vi "CRYSignal Generator.vi"(0 "Output Level(RMS)":dbl(knob)=10.0 caption="输出电平(RMS)" min=0.0 max=0.0 step=0.01 scale=0.0..1.0 scale format="%.1p", 1 "Manual":bool=TRUE, 2 "Output Device":u32, 5 "EQ":bool caption="均衡", 7 "Signal Path":i16(ring) caption="信号通道" items=["Left", "Right"], 9 "Execution control":T2={"interactive"=TRUE, "displayed"=TRUE, "in a seq"=FALSE}, 11 "Mute":bool=TRUE, 12 "Hardware in":string, 13 "Cancel":bool, 14 "Calibration in":string) -> (4 "Freq Out":dbl=1000.0 caption="Actual Freq" format="%.2f", 6 "Amp Out":dbl=0.01 caption="Actual level" format="%.2f", 8 "Sigal generator setup Out":string="%#_6p", 10 "Channel Out":u32, 15 "Canceled?":bool)   [LabVIEW 2013]
uses:
  Typedef Control/CRYWaveFile Information Typedef.ctl
  Typedef Control/CRYHardware Channel Info.ctl
  SubVI/CRYMisc vis settings global.vi
  Calibration/SubVI/CRYCal Global.vi
  CRYMainGlobal.vi
  Task Sequence/CRYProject Run Control Global.vi
  <vilib>/Analysis/NI_AALPro.lvlib
  CRYSound.dll
panel:
  in  "OK1":bool caption="ok"
  out "Play noise":sgl[](array[numeric]) caption="play noise"
  out "Out level":dbl
  in  "asio finished":bool
  out "wave data out":i32[](array[numeric])
  in  "Dur_asio":dbl=1.0 caption="檬" min=0.01 format="%.1f"
  in  "isMain":bool
  out "Gen_Index":i32
  in  "asio inited":bool
  in  "nTime_Count":u32 caption="%"
  in  "BuffAmount":u32
  out "Buffer Amount":i32
  in  "buf_index":u32 caption="%"
  in  "asio start":bool
  out "change flag":bool
  in  "Asio OCI":u32 caption="%"
  in  "ASIO AMP":dbl=0.1 caption="%" min=0.0 format="%.1f"
  in  "ASIO FS":dbl=0.1 caption="%" min=0.0 format="%.1f"
  in  "Device Name":string
  in  "Audio Driver":u16
  out "error out":errorcluster
  out "rms R":dbl
  out "rms L":dbl
  in  "Sel Channel":u16(ring) caption="Peak Unit" items=["Left", "Right"]
  out "Load Test":bool
  out "Configure Data":string
  out "Set Configure":bool
  out "lin2":bool
  out "lin1":bool
  out "log2":bool
  out "log1":bool
  out "Menu":bool=TRUE
  out "VI nID":i32
  out "Title nID":i32
  out "StateOut":bool=TRUE
  out "Error Output":errorcluster
  out "Wave L":dbl caption="Wave RMS" format="%0.2f"
  in  "ReMake Flg":bool
  in  "Play Sine Wave:":i32(slide) caption="播放正弦信号"
  out "noise":sgl[](array[numeric])
  out "Byte num":u32
  out "wave info":T1={"total number of samples/ch"=16, "total byte number"=2, "Time DBL"=0.0, "format str"="", "Time Str"="", "peak FSD"=0.0, "rms FSD"=0.0, "peak %FSD"=0.0, "rms %FSD"=0.0, "rms"=0.0, "Channel Number"=0, "rms L"=0.0, "rms R"=0.0}
  in  "Fs":u32=44100 caption="Sampling Frequency"
  in  "BitDepth":u32=16
  in  "ntaskID":u32
  in  "Max(Hz)":dbl=1.0 caption="最大(Hz)" min=1.0 step=1.0 format="%#.4p"
  in  "Min (Hz)":dbl=20.0 caption="最小(Hz)" min=1.0 max=20948.0 format="%#.4p"
  in  "Duration(s)":dbl=1.0 caption="时间(秒)" min=0.0 max=1000.0 step=1.0 format="%#.3p"
  out "Time":string
  out "stereo":string
  out "RMS":dbl format="%.4g"
  out "Peak":dbl caption="最大值" format="%_6f"
  in  "RMS Unit":u16(ring) items=["dB FSD", "%FSD"]
  in  "Peak Unit":u16(ring) items=["dB FSD", "%FSD"]
  in  "mute flash":bool
  in  "sine ol min":dbl=0.1 caption="V" min=0.0 format="%.3f"
  in  "sine ol max":dbl=0.1 caption="V" min=0.0 format="%.3f"
  in  "sine ol log":bool
  in  "wav ol log":bool
  in  "wav ol max":dbl=0.1 caption="V" min=0.0 format="%.3f"
  in  "wav ol min":dbl=0.1 caption="V" min=0.0 format="%.3f"
  in  "Duration":dbl=1.0 caption="秒" min=0.01 format="%.1f"
  in  "Signal Type":i32(ring) caption="信号类型" items=["正弦波", "wav", "粉红噪声", "白噪声"]
  in  "Wave path":string caption="波文件路径"
  in  "Wave play mode":i32(slide) caption="播放波文件"
  in  "n times":i32=1 caption="N次" min=1
  in  "wav level":dbl=0.1 caption="%" min=0.0 format="%.1f"
  in  "sine level":dbl=0.1 caption="V" min=0.0 format="%.3p"
  in  "freq lin/log":bool
  in  "level lin/log":bool
  in  "close at end":bool
  in  "dB":dbl=-40.0 min=-1000.0 max=1000.0 step=0.1 format="%.1f"
  out "unit2":string="V"
  out "Error":u32
  in  "Sweep Rate":dbl=1.0 caption="Octave/s" min=0.1 step=0.01 format="%.2f"
  in  "Quadrature":bool
  in  "Sensitivity":dbl=1.0 min=0.1 step=0.01 format="%.6f"
  in  "Frequency":dbl(knob)=1000.0 caption="频率" min=10.0 max=20948.0 step=1.0 scale=20.0..20000.0
  out "mute border":bool
  in  "cont":bool=TRUE
  in  "Vp Out":dbl=2.6 min=0.1 step=0.01 format="%.2f"
  out "unit1":string="Hz"
  in  "Browse":bool
  in  "start":bool
  in  "stop":bool
  in  "OK":bool caption="ok"
  in  "cancel2":bool
  in  "1 kHz":bool
  in  "Equalization Out":cluster{"Hz":dbl, dbl, "Deg":dbl}[](array[cluster])=[{"Hz"=1.0, 1.0, "Deg"=0.0}, {"Hz"=20000.0, 1.0, "Deg"=0.0}] {"Deg" format="%.2f"; "?" format="%.2f"; "Hz" format="%.2f"}
  in  "dB ref.":dbl=1.0 min=0.01 step=0.01 format="%.6f"
  in  "prefix Out":string
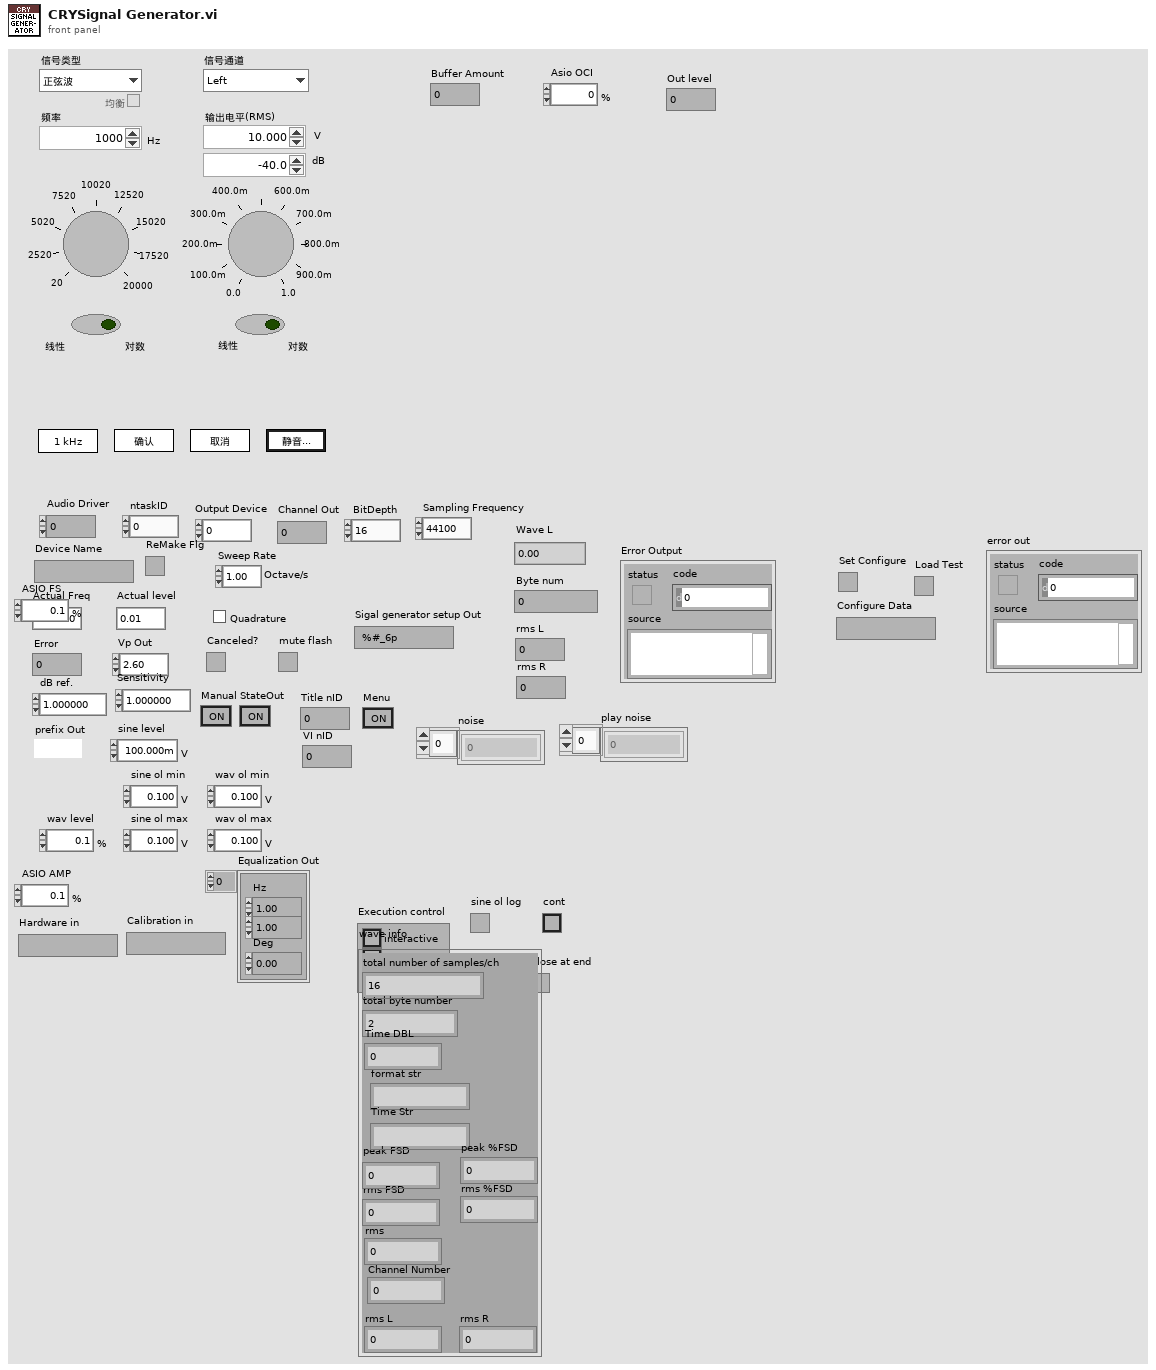
[diagram p1: front panel]
types:
  T1 = typedef "CRYWaveFile Information Typedef.ctl" = cluster{"total number of samples/ch":u32, "total byte number":u32, "Time DBL":dbl, "format str":string, "Time Str":string, "peak FSD":dbl, "rms FSD":dbl, "peak %FSD":dbl, "rms %FSD":dbl, "rms":dbl, "Channel Number":u16, "rms L":dbl, "rms R":dbl}
  T2 = cluster{"interactive":bool, "displayed":bool, "in a seq":bool}
  T3 = enum32{"Invalid", "Default", "Floating", "Floating/Auto-Hide", "Modal"}
  T4 = cluster{"wav play mode":i32, "start":bool, "Output Level(RMS)":dbl, "Output Level(dB)":dbl, "level lin/log":bool}
  T5 = cluster{"wav init":bool, "halt now":bool, "exit":bool, "dll done":bool, "called":bool, "changed":bool, "Hardware":i32}
  T6 = typedef "CRYCalibration All Cluster.ctl" = cluster{"Calibration 2D":T7[], "Help":string, "Tab Value":i32, "Input Signal Type":string, "Output Signal Type":string}
  T7 = typedef "CRYCalibration 2DCluster.ctl" = cluster{"Calibration":T8, "Corr Curve":T9, "EQ Curve":T9, "Sens Curve":T9}
  T8 = typedef "CRYCalibration Cluster.ctl" = cluster{"Calibration Step Name":string, "Device":string, "Correction Curve Name":string, "Equalization Curve Name":string, "Sensitivity Curve Name":string, "Corr Folder and File":string, "EQ Folder and File":string, "Sens Folder and File":string, "Corr Step size":u16, "EQ Step size":u16, "Input":bool, "Last Cal Date (sec)":timestamp, "Cha Name":string, "Corr Curve Found":bool, "EQ Curve Found":bool, "Sens Curve Found":bool, "Signal Type":string, "Calibrated Device":string, "Hz":u32}
  T9 = typedef "CRYData Cluster.ctl" = cluster{"Name":string, "Curve":cluster{"x":dbl, "y":dbl, "z":dbl}[], "X data":u16, "Y data":u16, "Z data":u16, "X axis":u16, "Y axis":u16, "Z axis":u16, "X unit":string, "Y unit":string, "Z unit":string, "X dB ref":dbl, "Y dB ref":dbl, "Z dB ref":dbl, "single val":bool, "protected":bool, "display X":bool, "display Y":bool, "display Z":bool, "Test Info":string, "Step No.":i32, "Plot Settings":cluster{"Color":u32, "Interpolation":u8, "Point Style":u8, "Line Style":u8, "Point Color":u32, "Line Width":u8, "Bar Plot Style":u8, "Fill To":i16}, "AutoProtect":bool}
  T10 = enum8{"Enabled", "Disabled", "Disabled and Grayed Out"}
  T11 = cluster{"gen'r mode":i32, "frequency":u32, "output level":dbl, "wave path":string, "wav play mode":i32, "duration":dbl, "n times":i32, "channel":i32, "wav level":dbl, "EQ":bool, "f knob log":bool, "f knob low":dbl, "f knob high":dbl, "ol knob log":bool, "ol knob low":dbl, "ol knob high":dbl, "Lin Display Prefs":string, "dB Display Prefs":string, "Duration noise":dbl, "Min freq noise":dbl, "Max freq noise":dbl, "Signal Type":string, "Play Sine Wave":i32}
  T12 = typedef "CRYHardware Channel Info.ctl" = cluster{"ID":i32, "Name":string, "Digital":bool, "Input":bool, "Device Name":string, "Hardware Ch ID":u8, "Vmax (V)":dbl, "Latency (samples)":dbl, "Sampling Rate (Hz)":u32, "Bit Depth":u32, "Anti-aliasing Factor (%fs)":sgl, "DAQmx Channel":tag, "term config":i32, "Coupling":i32, "IEPE en":bool, "ASIOChannel Name":string, "Audio Driver":u16, "ASIOChannel Index":u8}
  T13 = enum16{"sine", "cosine", "triangle", "square", "sawtooth", "increasing ramp", "decreasing ramp"}
  T14 = cluster{"Wave play mode":i32, "start":bool, "Output Level(RMS)":dbl, "dB":dbl, "level lin/log":bool}
  T15 = cluster{"Level Type":u16, "Vp Out":dbl, "Output Level(RMS)":dbl}
  T16 = cluster{"Gen Idx":i32, "Chn Idx":i32, "Data":sgl[]}[]
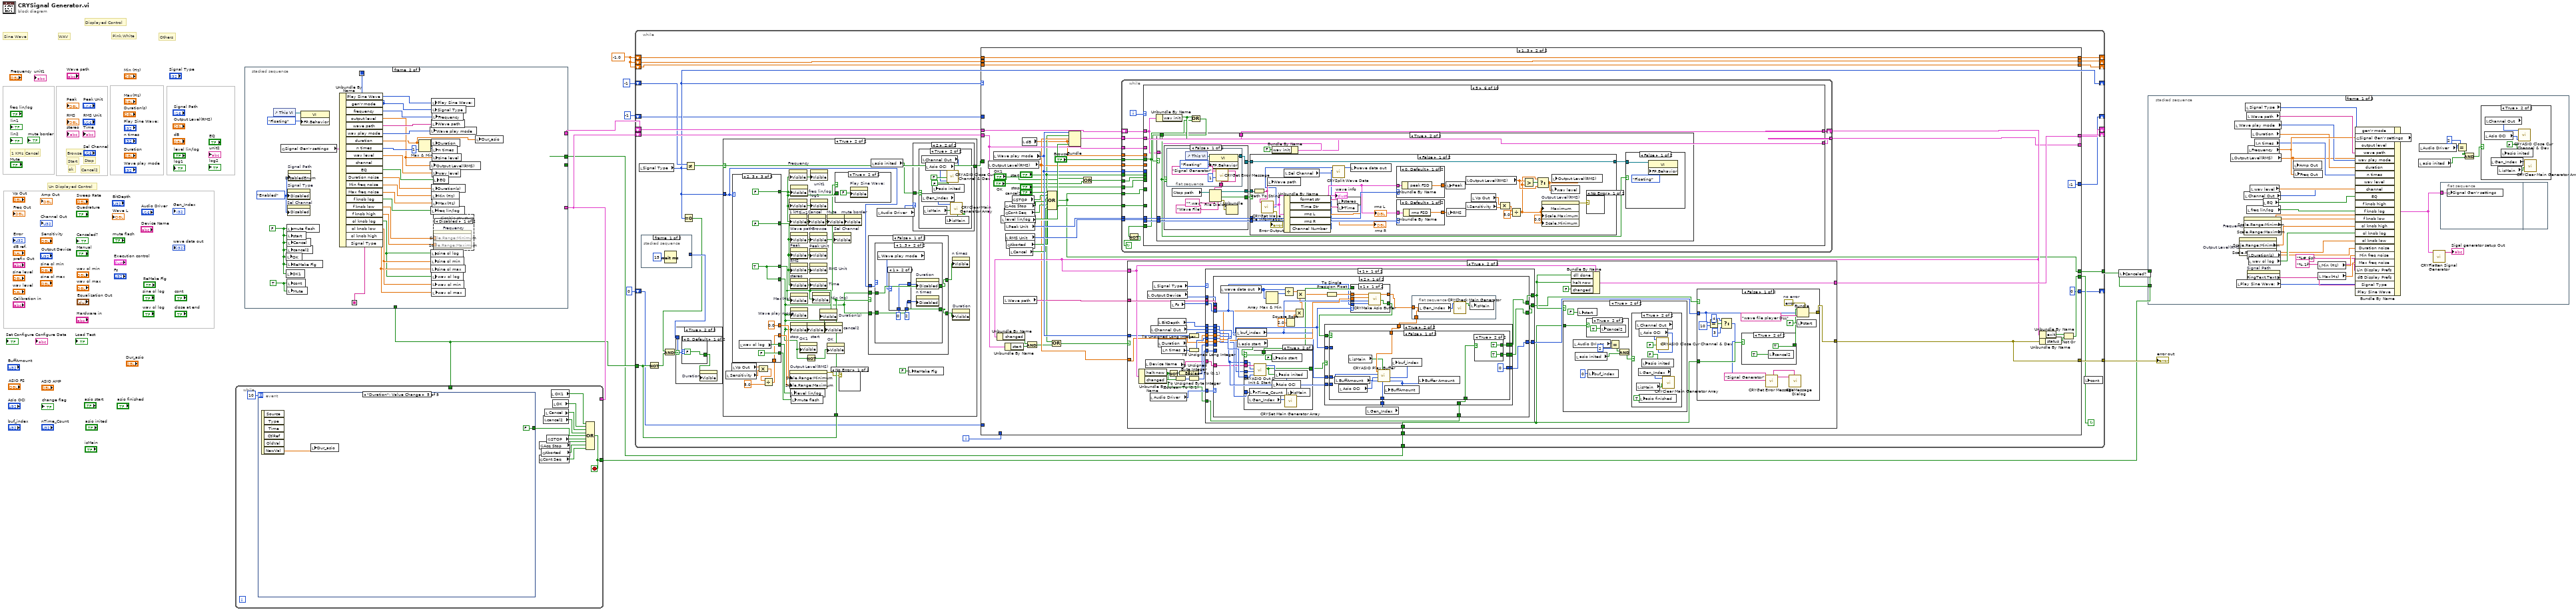
[diagram p0: block diagram]
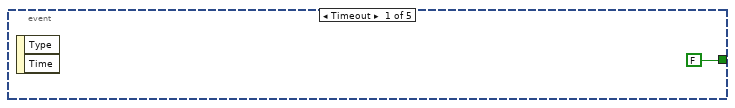
[diagram p2: hidden frame]
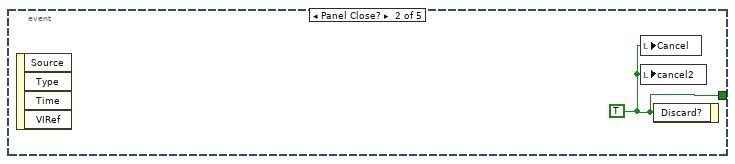
[diagram p3: hidden frame]
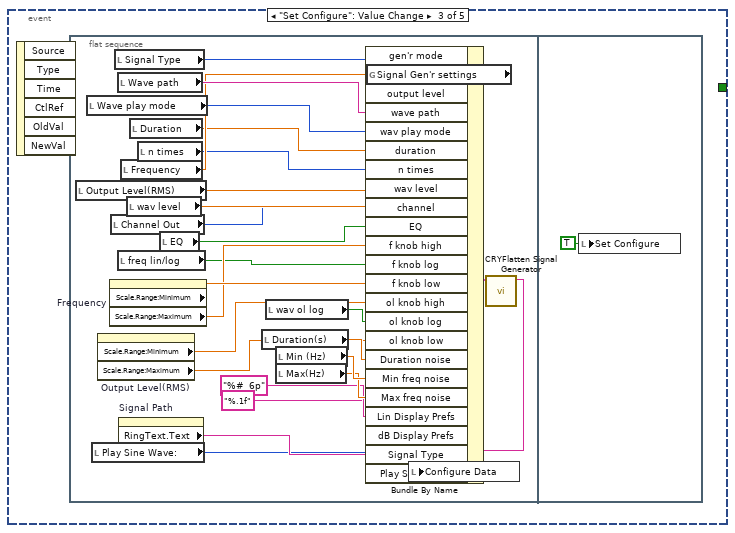
[diagram p4: hidden frame]
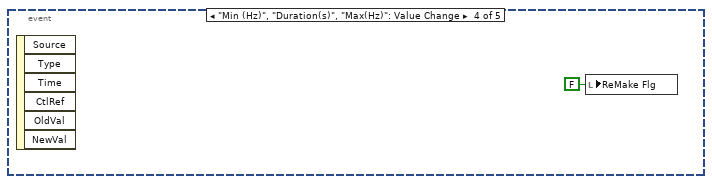
[diagram p5: hidden frame]
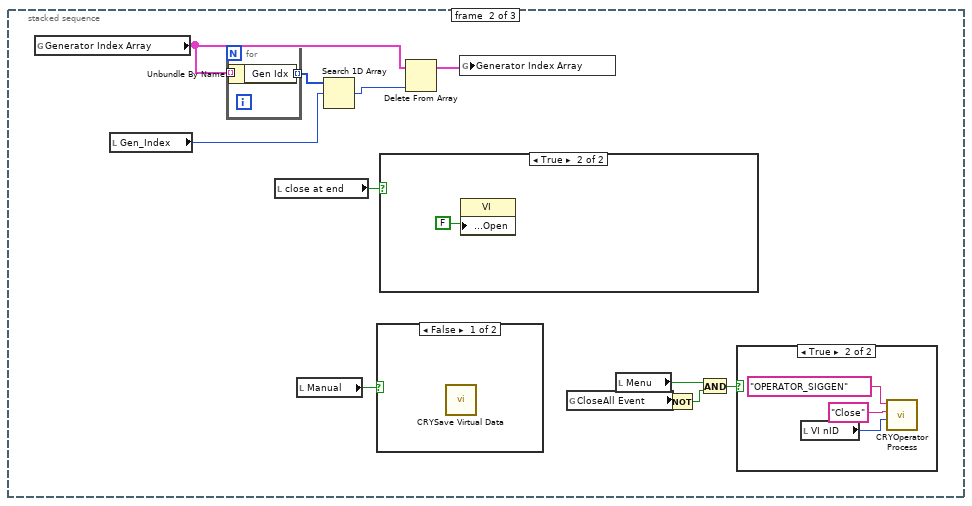
[diagram p7: hidden frame]
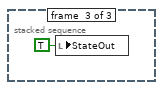
[diagram p11: hidden frame]
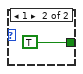
[diagram p13: hidden frame]
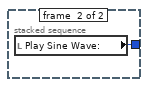
[diagram p14: hidden frame]
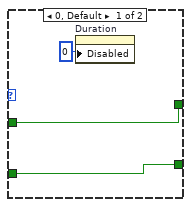
[diagram p19: hidden frame]
diagram:
  w1 = -1.0 ("Frequency")
  # "Others"
  # "WAV"
  # "Pink,White"
  # "Sine Wave"
  # "Un Displayed Control"
  # "Displayed Control"
  # "ok"
  # "Cancel2"
  # "Stop"
  # "Start"
  # "Browse"
  # "Cancel"
  # "1 KHz"
  n1 = stacked-sequence {
    seq-local: [_ w45 _ _ _ _ _] -> [_ _ _ w124 _ _ _]
    seq-local: [_ w41 _ _ _ _ _] -> [_ _ w66 _ _ _ _]
    tunnel: [_ _ _ w129 _ _ _] -> _
    tunnel: [_ _ _ w121 _ _ _] -> w4
    tunnel: [_ _ _ _ _ w170 _] -> w9
    tunnel: [_ _ _ _ _ T4 {"wav play mode"=-1, "start"=FALSE, "Output Level(RMS)"=0.0, "Output Level(dB)"=0.0, "level lin/log"=FALSE} _] -> w8
    tunnel: [_ _ _ w125 _ _ _] -> w7
    frame #0 {
      w16 = FALSE ("StateOut")
      n2 = call "CRYMake Generator Index.vi"() -> ("Gen_Index"=w12:i32)  [unwired: 11 in]
      n3 = local write "Set Configure"(w16) -> ()
      n4 = global read "CRYMisc vis settings global.vi" "Menu?"() -> (w21:bool)
      "Menu" <- w21
      n5 = local write "Gen_Index"(w12) -> ()
      n6 = call "CRYGet Window Title Message.vi"("No"=0 ("Error No"), "Kind"="Signal Generator") -> ("Multibyte String"=w19:string)  [unwired: 4 in, 5 out]
      n7 = case shown="True" w21 {
        tunnel: w19 -> [w24 w31]
        tunnel: [w24 w30] -> w18
        tunnel: [w23 w25] -> w13
        frame False {
          n8 = control-ref of="This VI"() -> (w22:refnum<vi>)
          n9 = call "CRYSet Signal Generator Front Panel.vi"("Vi Ref in"=w22) -> ()  [unwired: 10 in, 1 out]
          n10 = local read "Calibration in"() -> (w23:string)
        }
        frame True {
          n11 = global read "CRYMisc vis settings global.vi" "Execution control"() -> (w27:T2)
          n12 = global read "CRYMisc vis settings global.vi" "Temp Title nID"() -> (w32:i32)
          "Title nID" <- w32
          n13 = global read "CRYMisc vis settings global.vi" "Temp VI nID"() -> (→"VI nID":i32)
          n14 = global read "CRYMisc vis settings global.vi" "Manual"() -> (w34:bool)
          n15 = global read "CRYMisc vis settings global.vi" "Mute"() -> (w35:bool)
          n16 = call "CRYGet Current HC Steps.vi"() -> ("Calibration setup flattened Out"=w25:string, "Hardware setup flattened Out"=w26:string)  [unwired: 10 out]
          n17 = local write "Calibration in"(w25) -> ()
          n18 = local write "Hardware in"(w26) -> ()
          n19 = Number To Decimal String(number=w32) -> (decimal integer string=w29:string)  [unwired: 1 in]
          n20 = local write "Execution control"(w27) -> ()
          n21 = local write "Manual"(w34) -> ()
          n22 = local write "Mute"(w35) -> ()
          n23 = Concatenate Strings(w31, "-" ("string"), w29) -> (w30:string)
        }
      }
      n24 = property class="VI"("Front Panel.Title"=w18) -> ()  [unwired: 2 in, 2 out]
      n25 = call "CRYUnflatten Calibration 2D.vi"("Flattened Calibration"=w13) -> ("Calibration Step Out"=w14:T6)  [unwired: 8 in, 2 out]
      n26 = call "CRYGet Calibrated Device Name.vi"("Calibration"=w14) -> ("O_Signal Type Out"=w15:string[])  [unwired: 7 in, 7 out]
      n27 = property on="Signal Path" class="Ring (strict)"("Strings []"=w15) -> ()  [unwired: 2 in, 2 out]
      "StateOut" <- w16
    }
    frame #1 {
      w37 = T10."Enabled" ("Disabled")
      w44 = TRUE ("cont")
      w36 = FALSE ("Mute")
      n28 = control-ref of="This VI"() -> (w43:refnum<vi>)
      n29 = global read "CRYMisc vis settings global.vi" "Signal Gen'r settings"() -> (w53:T11)
      n30 = local write "OK"(w36) -> ()
      n31 = local write "OK1"(w36) -> ()
      n32 = local write "mute flash"(w36) -> ()
      n33 = local write "start"(w36) -> ()
      n34 = local write "Cancel"(w36) -> ()
      n35 = local write "cancel2"(w36) -> ()
      n36 = local write "ReMake Flg"(w36) -> ()
      n37 = local write "cont"(w44) -> ()
      n38 = local write "Mute"(w44) -> ()
      n39 = property on="Signal Type" class="Ring (strict)"("Disabled"=w37) -> ()  [unwired: 2 in, 2 out]
      n40 = property on="Sel Channel" class="Ring (strict)"("Disabled"=w37) -> ()  [unwired: 2 in, 2 out]
      n41 = property on="Signal Path" class="Ring (strict)"("DisabledEnum"=w37) -> ()  [unwired: 2 in, 2 out]
      n42 = property class="VI"(reference=w43, "FP.Behavior"=T3."Floating" ("Front Panel Window:Behavior")) -> ()  [unwired: 1 in, 2 out]
      n43 = Unbundle By Name(w53) -> ("Play Sine Wave"=w40:i32, "gen'r mode"=w45:i32, "frequency"=w58:u32, "output level"=w46:dbl, "wave path"=w60:string, "wav play mode"=w59:i32, "duration"=w38:dbl, "n times"=w61:i32, "wav level"=w57:dbl, "EQ"=w56:bool, "Duration noise"=w39:dbl, "Min freq noise"=w55:dbl, "Max freq noise"=w54:dbl, "f knob log"=w47:bool, "f knob low"=w48:dbl, "f knob high"=w49:dbl, "ol knob log"=w50:bool, "ol knob low"=w52:dbl, "ol knob high"=w51:dbl, "Signal Type"=w41:string)  [unwired: 1 out]
      n44 = Max & Min(x=1, y=w61) -> (max(x,y)=w62:i32)  [unwired: 1 out]
      n45 = local write "Wave play mode"(w59) -> ()
      n46 = local write "Output Level(RMS)"(w46) -> ()
      n47 = local write "freq lin/log"(w47) -> ()
      n48 = local write "sine ol log"(w50) -> ()
      n49 = local write "sine ol min"(w52) -> ()
      n50 = local write "sine ol max"(w51) -> ()
      n51 = local write "Play Sine Wave:"(w40) -> ()
      n52 = local write "Signal Type"(w45) -> ()
      n53 = local write "wav ol log"(w50) -> ()
      n54 = local write "wav ol min"(w52) -> ()
      n55 = local write "Wave path"(w60) -> ()
      n56 = local write "Duration"(w38) -> ()
      n57 = local write "Duration(s)"(w39) -> ()
      n58 = local write "Min (Hz)"(w55) -> ()
      n59 = local write "wav ol max"(w51) -> ()
      n60 = local write "Frequency"(w58) -> ()
      n61 = local write "n times"(w62) -> ()
      n62 = local write "sine level"(w46) -> ()
      n63 = local write "wav level"(w57) -> ()
      n64 = local write "Max(Hz)"(w54) -> ()
      n65 = local write "EQ"(w56) -> ()
      n66 = disable-structure shown="Disabled" {
        disable-tunnel: w49 -> [w65 _]
        disable-tunnel: w48 -> [w64 _]
        frame Disabled {
          n67 = property on="Frequency" class="Knob (strict)"("Scale.Range:Minimum"=w64, "Scale.Range:Maximum"=w65) -> ()  [unwired: 2 in, 2 out]
        }
        frame Enabled {
        }
      }
      n68 = local write "Dur_asio"(w38) -> ()
    }
    frame #2 {
      # "Initialize"
      n69 = local read "Manual"() -> (w67:bool)
      n70 = case shown="False" w67 {
        tunnel: w66 -> [w78 _]
        frame False {
          n71 = global read "CRYCal Global.vi" "Calibrate"() -> (w73:bool)
          n72 = local read "Calibration in"() -> (w74:string)
          n73 = local read "Hardware in"() -> (w75:string)
          n74 = case shown="False" w73 {
            tunnel: w78 -> [w89 _]
            tunnel: [w92 w107] -> w77
            tunnel: w75 -> [w91 w109]
            tunnel: w74 -> [w90 w108]
            tunnel: [w86 w106] -> w76
            frame False {
              n75 = call "CRYGet Hardware Info From Signal Type.vi"("Calibration In"=w90, "Hardware In"=w91, "Signal Type"=w89, "In/Out?"=FALSE) -> ("Exist?"=w94:bool, "Channel Info Out"=w93:T12)  [unwired: 5 in, 1 out]
              n76 = property on="Signal Path" class="Ring (strict)"() -> ("Strings []"=w88:string[])  [unwired: 2 in, 2 out]
              n77 = case shown="False" w94 {
                tunnel: w93 -> [_ w102]
                tunnel: [w97 w102] -> w92
                tunnel: w91 -> [w100 _]
                tunnel: w90 -> [w99 _]
                tunnel: w89 -> [_ w101]
                tunnel: [w96 w101] -> w87
                frame False {
                  w96 = "Direct Out 1" ("Signal Type")
                  n78 = call "CRYGet Hardware Info From Signal Type.vi"("Calibration In"=w99, "Hardware In"=w100, "Signal Type"=w96, "In/Out?"=FALSE) -> ("Channel Info Out"=w97:T12)  [unwired: 5 in, 2 out]
                }
                frame True {
                }
              }
              n79 = Search 1D Array(1D array=w88, element=w87) -> (index of element=w86:i32)  [unwired: 1 in]
            }
            frame True {
              n80 = global read "CRYCal Global.vi" "Signal Type Out"() -> (w106:u16)
              n81 = property on="Signal Path" class="Ring (strict)"() -> ("Strings []"=w105:string[])  [unwired: 2 in, 2 out]
              n82 = Index Array(array=w105, index=w106) -> (element=w103:string)
              n83 = call "CRYGet Hardware Info From Signal Type.vi"("Calibration In"=w108, "Hardware In"=w109, "Signal Type"=w103, "In/Out?"=FALSE) -> ("Channel Info Out"=w107:T12)  [unwired: 5 in, 2 out]
            }
          }
          n84 = local write "buf_index"(u32 0 ("buf_index")) -> ()
          n85 = Unbundle By Name(w77) -> ("ID"=w79:i32, "Hardware Ch ID"=w69:u8, "Vmax (V)"=w72:dbl, "Sampling Rate (Hz)"=w80:u32, "Bit Depth"=w81:u32, "Audio Driver"=w68:u16, "Device Name"=w71:string)
          n86 = local write "Signal Path"(w76) -> ()
          n87 = local write "Device Name"(w71) -> ()
          n88 = local write "Output Device"(w79) -> ()
          n89 = local write "Channel Out"(w69) -> ()
          n90 = local write "BitDepth"(w81) -> ()
          n91 = local write "Vp Out"(w72) -> ()
          n92 = local write "Fs"(w80) -> ()
          n93 = case shown="0, Default" w68 {
            tunnel: w69 -> [_ w85]
            frame 0, Default {
              n94 = local read "Gen_Index"() -> (w83:i32)
              n95 = call "CRYUpdate Generator Index.vi"("Chn Idx"=-1, "Gen_Index"=w83) -> ()  [unwired: 9 in]
            }
            frame 2 {
              n96 = local read "Gen_Index"() -> (w84:i32)
              n97 = call "CRYUpdate Generator Index.vi"("Chn Idx"=w85, "Gen_Index"=w84) -> ()  [unwired: 9 in]
            }
          }
          n98 = local write "Audio Driver"(w68) -> ()
        }
        frame True {
          w110 = T12[] [{"ID"=1, "Name"="Left", "Digital"=FALSE, "Input"=FALSE, "Device Name"="Card", "Hardware Ch ID"=0, "Vmax (V)"=2.6, "Latency (samples)"=67.0, "Sampling Rate (Hz)"=44100, "Bit Depth"=16, "Anti-aliasing Factor (%fs)"=44100.0, "DAQmx Channel"="", "term config"=0, "Coupling"=0, "IEPE en"=FALSE, "ASIOChannel Name"="", "Audio Driver"=0, "ASIOChannel Index"=0}, {"ID"=1, "Name"="Right", "Digital"=FALSE, "Input"=FALSE, "Device Name"="Card", "Hardware Ch ID"=1, "Vmax (V)"=2.6, "Latency (samples)"=67.0, "Sampling Rate (Hz)"=44100, "Bit Depth"=16, "Anti-aliasing Factor (%fs)"=44100.0, "DAQmx Channel"="", "term config"=0, "Coupling"=0, "IEPE en"=FALSE, "ASIOChannel Name"="", "Audio Driver"=0, "ASIOChannel Index"=0}] ("I_channel Info Out")
          n99 = call "CRYGet Channel Array.vi"("Channel Array"=w110) -> ("O_Channel Name Out"=w114:string[])  [unwired: 10 out]
          n100 = property on="Signal Path" class="Ring (strict)"("Strings []"=w114) -> ()  [unwired: 2 in, 2 out]
          n101 = Index Array(array=w110, index=1) -> (element=w120:T12)
          n102 = Unbundle By Name(w120) -> ("ID"=w118:i32, "Hardware Ch ID"=w119:u8)
          n103 = local write "Output Device"(w118) -> ()
          n104 = property on="Play Sine Wave:" class="Slide (strict)"("Visible"=FALSE) -> ()  [unwired: 2 in, 2 out]
          n105 = local write "Channel Out"(w119) -> ()
          n106 = local write "Vp Out"(2.6 ("Vmax (V)")) -> ()
          n107 = local write "BitDepth"(u32 16 ("BitDepth")) -> ()
          n108 = global write "CRYMainGlobal.vi" "STOP"(FALSE ("STOP")) -> ()
          n109 = local write "Fs"(u32 44100 ("Sampling Frequency")) -> ()
        }
      }
    }
    frame #3 {
      # "(formerly always displayed panel in continuous-play mode)"
      n110 = local read "Execution control"() -> (w127:T2)
      n111 = local read "Wave play mode"() -> (w126:i32)
      n112 = Unbundle By Name(w127) -> ("in a seq"=w121:bool, "interactive"=w125:bool, "displayed"=w132:bool)
      n113 = Equal To 0?(x=w126) -> (x = 0?=w128:bool)
      n114 = Greater Than 0?(x=w124) -> (x > 0?=w123:bool)
      n115 = case shown="False" w121 {
        frame False {
          w133 = 0 items=["Continuously", "for Duration"] ("Play Sine Wave:")
          n116 = local write "Play Sine Wave:"(w133) -> ()
        }
        frame True {
        }
      }
      n117 = property class="VI"() -> ("Front Panel Window:Open"=w122:bool)  [unwired: 2 in, 2 out]
      n118 = case shown="False" w123 {
        tunnel: w121 -> [w135 w136]
        frame False {
          n119 = Not(x=w135) -> (.not. x?=w134:bool)
          n120 = local write "Mute"(w134) -> ()
        }
        frame True {
          n121 = local write "start"(w136) -> ()
        }
      }
      n122 = Compound Arithmetic op=OR(invert w121, w128) -> (w129:bool)
      n123 = Or(x=w125, y=w132) -> (x .or. y?=w131:bool)
      n124 = Compound Arithmetic op=AND(w131, invert w122) -> (w130:bool)
      n125 = case shown="True" w131 {
        tunnel: w131 -> [_ w137]
        tunnel: w130 -> [_ _]
        frame False {
        }
        frame True {
          n126 = flat-sequence {
            tunnel: w137 -> [w138]
            frame #0 {
              n127 = property class="VI"("Front Panel Window:Open"=w138) -> ()  [unwired: 2 in, 2 out]
            }
            frame #1 {
              n128 = Wait (ms)(milliseconds to wait=u32 150) -> ()  [unwired: 1 out]
            }
          }
        }
      }
      n129 = local write "close at end"(w130) -> ()
    }
    frame #4 {
      n130 = local read "Manual"() -> (w140:bool)
      n131 = case shown="False" w140 {
        frame False {
          n132 = property on="Signal Path" class="Ring (strict)"() -> ("RingText.Text"=w147:string)  [unwired: 2 in, 2 out]
          n133 = call "CRYGet Current Calibration Info.vi"("Is Input?"=FALSE, "Signal Type Name"=w147) -> ("Calibration All Cluster"=w146:T7)  [unwired: 9 out]
          n134 = Unbundle By Name(w146) -> ("EQ Curve"=w154:T9, "Sens Curve"=w156:T9)
          n135 = Unbundle By Name(w156) -> ("Curve"=w158:cluster{"x":dbl, "y":dbl, "z":dbl}[], "Y unit"=w142:string, "Y dB ref"=w149:dbl)
          n136 = Unbundle By Name(w154) -> ("Curve"=w155:cluster{"x":dbl, "y":dbl, "z":dbl}[])  [unwired: 1 out]
          n137 = global read "CRYCal Global.vi" "Calibrate"() -> (w152:bool)
          n138 = local write "Equalization Out"(w155) -> ()
          n139 = Reverse String(1:w142) -> (0:w145:string)
          n140 = Index Array(array=w158) -> (element=w157:cluster{"x":dbl, "y":dbl, "z":dbl})  [unwired: 1 in]
          n141 = Unbundle By Name(w157) -> ("y"=w151:dbl)
          n142 = case shown="False" w152 {
            tunnel: w151 -> [w160 _]
            tunnel: w149 -> [w159 _]
            tunnel: [w160 w162] -> w150
            tunnel: [w159 1.0 ("Y dB ref")] -> w148
            frame False {
            }
            frame True {
              n143 = global read "CRYCal Global.vi" "Sens Out"() -> (w162:dbl)
            }
          }
          n144 = Match Pattern(string=w145, regular expression="/" ("search char (-)")) -> (after substring=w143:string)  [unwired: 1 in, 3 out]
          n145 = Reverse String(1:w143) -> (0:w141:string)
          n146 = local write "dB ref."(w148) -> ()
          n147 = local write "Sensitivity"(w150) -> ()
          n148 = local write "unit2"(w141) -> ()
        }
        frame True {
          w165 = 0 items=["Sine Wave", "WAV", "Pink Noise", "White Noise"] ("Signal Type")
          n149 = local write "Signal Type"(w165) -> ()
          n150 = local write "Sensitivity"(1.0 ("Sensitivity")) -> ()
          n151 = property class="DigNum (strict)"("Value"=0.2) -> ()  [unwired: 2 in, 2 out]
          n152 = property class="DigNum (strict)"("Value"=1000.0) -> ()  [unwired: 2 in, 2 out]
          n153 = local write "dB ref."(1.0 ("dB Ref Out")) -> ()
        }
      }
    }
    frame #5 {
      n154 = local read "Signal Type"() -> (w169:i32)
      n155 = Not Equal To 0?(x=w169) -> (x != 0?=w172:bool)
      n156 = case shown="True" w172 {
        tunnel: T5 {"wav init"=TRUE, "halt now"=FALSE, "exit"=FALSE, "dll done"=FALSE, "called"=FALSE, "changed"=FALSE, "Hardware"=-1} -> [w173 w177]
        tunnel: [w173 w176] -> w170
        frame False {
        }
        frame True {
          n157 = Bundle By Name(cluster=w177, "called"=TRUE ("Bundle Element"), "Hardware"=-1) -> (w176:T5)
        }
      }
    }
    frame #6 {
      n158 = local read "Sensitivity"() -> (w182:dbl)
      n159 = local read "dB ref."() -> (w180:dbl)
      n160 = Less Or Equal To 0?(x=w182) -> (x <= 0?=w181:bool)
      n161 = Less Or Equal To 0?(x=w180) -> (x <= 0?=w179:bool)
      n162 = local write "Load Test"(TRUE ("Load Test")) -> ()
      n163 = case shown="True" w181 {
        frame False {
        }
        frame True {
          n164 = local write "Sensitivity"(1.0 ("Sensitivity")) -> ()
        }
      }
      n165 = case shown="True" w179 {
        frame False {
        }
        frame True {
          n166 = local write "dB ref."(1.0 ("dB ref.")) -> ()
        }
      }
    }
  }
  n167 = while {
    tunnel: w8 -> [_]
    tunnel: [w186] -> w3
    tunnel: w7 -> [_]
    stop <- w186 stop-if-true
    n168 = event shown="[4] \"Duration\": Value Change" {
      selector: _ -> [_ _ _ _ _]
      dyn-events: _ -> [_ _ _ _ _]
      timeout: 10 -> [_ _ _ _ _]
      tunnel: [FALSE ("Discard?") w197 _ _ FALSE ("Discard?")] -> w194
      event Timeout {
        n169 = event-data() -> ()  [unwired: 3 out]
      }
      event Panel Close? {
        w197 = TRUE ("Discard?")
        n170 = event-data() -> ()  [unwired: 5 out]
        n171 = local write "Cancel"(w197) -> ()
        n172 = local write "cancel2"(w197) -> ()
        n173 = event-data("Discard?"=w197) -> ()  [unwired: 1 in, 1 out]
      }
      event "Set Configure": Value Change {
        n174 = event-data() -> ()  [unwired: 7 out]
        n175 = flat-sequence {
          frame #0 {
            n176 = local read "Output Level(RMS)"() -> (w201:dbl)
            n177 = local read "Wave play mode"() -> (w220:i32)
            n178 = local read "Play Sine Wave:"() -> (w199:i32)
            n179 = property on="Output Level(RMS)" class="Knob (strict)"() -> ("Scale.Range:Minimum"=w208:dbl, "Scale.Range:Maximum"=w207:dbl)  [unwired: 2 in, 2 out]
            n180 = property on="Frequency" class="Knob (strict)"() -> ("Scale.Range:Minimum"=w217:dbl, "Scale.Range:Maximum"=w216:dbl)  [unwired: 2 in, 2 out]
            n181 = local read "Channel Out"() -> (w203:u32)
            n182 = local read "Signal Type"() -> (w204:i32)
            n183 = local read "Wave path"() -> (w222:string)
            n184 = local read "freq lin/log"() -> (w206:bool)
            n185 = property on="Signal Path" class="Ring (strict)"() -> ("RingText.Text"=w202:string)  [unwired: 2 in, 2 out]
            n186 = local read "Frequency"() -> (w221:dbl)
            n187 = local read "wav level"() -> (w205:dbl)
            n188 = local read "Duration"() -> (w219:dbl)
            n189 = local read "n times"() -> (w218:i32)
            n190 = local read "EQ"() -> (w211:bool)
            n191 = local read "Duration(s)"() -> (w214:dbl)
            n192 = local read "wav ol log"() -> (w215:bool)
            n193 = local read "Min (Hz)"() -> (w213:dbl)
            n194 = local read "Max(Hz)"() -> (w212:dbl)
            n195 = global read "CRYMisc vis settings global.vi" "Signal Gen'r settings"() -> (w200:T11)
            n196 = Bundle By Name(cluster=w200, "gen'r mode"=w204, "frequency"=w221, "output level"=w201, "wave path"=w222, "wav play mode"=w220, "duration"=w219, "n times"=w218, "wav level"=w205, "channel"=w203, "EQ"=w211, "f knob high"=w216, "f knob log"=w206, "f knob low"=w217, "ol knob high"=w208, "ol knob log"=w215, "ol knob low"=w207, "Duration noise"=w214, "Min freq noise"=w213, "Max freq noise"=w212, "Lin Display Prefs"="%#_6p", "dB Display Prefs"="%.1f", "Signal Type"=w202, "Play Sine Wave"=w199) -> (w223:T11)
            n197 = call "CRYFlatten Signal Generator.vi"("Signal Gen'r settings"=w223) -> ("Flat Signal Gen'r settings"=w198:string)  [unwired: 10 out]
            n198 = local write "Configure Data"(w198) -> ()
          }
          frame #1 {
            n199 = local write "Set Configure"(TRUE ("Set Configure")) -> ()
          }
        }
      }
      event "Min (Hz)", "Duration(s)", "Max(Hz)": Value Change {
        n200 = event-data() -> ()  [unwired: 7 out]
        n201 = local write "ReMake Flg"(FALSE ("ReMake Flg")) -> ()
      }
      event "Duration": Value Change {
        n202 = event-data() -> ("NewVal"=w227:dbl)  [unwired: 6 out]
        n203 = local write "Dur_asio"(w227) -> ()
      }
    }
    n204 = global read "CRYProject Run Control Global.vi" "Cont Seq"() -> (w187:bool)
    n205 = global read "CRYMainGlobal.vi" "Acq Stop"() -> (w189:bool)
    n206 = global read "CRYProject Run Control Global.vi" "Aborted"() -> (w188:bool)
    n207 = local read "cancel2"() -> (w192:bool)
    n208 = local read "Cancel"() -> (w193:bool)
    n209 = global read "CRYMainGlobal.vi" "STOP"() -> (w191:bool)
    n210 = local read "OK1"() -> (w185:bool)
    n211 = local read "OK"() -> (w190:bool)
    n212 = Compound Arithmetic op=OR(w185, w190, w193, w192, w194, w191, w189, w188, w187) -> (w186:bool)
  }
  n213 = while {
    tunnel: [w255] -> w10
    shift-right: [w254] -> _
    shift-left: w8 -> [w253]
    shift-right: [w251] -> _
    shift-left: w9 -> [w252]
    tunnel: [w250] -> w5
    shift-right: [w245] -> _
    shift-left: -1 ("Signal Type") -> [w248]
    tunnel: w4 -> [w241]
    tunnel: w7 -> [w240]
    shift-right: [w237] -> _
    shift-left: i16 -1 ("Channel") -> [w238]
    shift-right: [w235] -> _
    shift-left: 0 ("Buffer Amount") -> [w234]
    shift-right: [w230] -> _
    shift-left: w1 -> [w233]
    shift-right: [w229] -> _
    shift-left: w1 -> [w232]
    shift-right: [w228] -> _
    shift-left: w1 -> [w231]
    i -> [w239]
    stop <- w249 continue-if-true
    n214 = local read "Signal Type"() -> (w245:i32)
    n215 = stacked-sequence {
      tunnel: [_ w261] -> w246
      frame #0 {
        n216 = Wait (ms)(milliseconds to wait=u32 15) -> ()  [unwired: 1 out]
      }
      frame #1 {
        n217 = local read "Play Sine Wave:"() -> (w261:i32)
      }
    }
    n218 = Not(x=w240) -> (.not. x?=w242:bool)
    n219 = Equal To 0?(x=w245) -> (x = 0?=w243:bool)
    n220 = And(x=w243, y=w242) -> (x .and. y?=w244:bool)
    n221 = case shown="True" w244 {
      tunnel: w246 -> [_ w257]
      frame False {
      }
      frame True {
        n222 = case shown="0, Default" w257 {
          tunnel: [FALSE TRUE] -> w256
          frame 0, Default {
          }
          frame 1 {
          }
        }
        n223 = property on="Duration" class="DigNum (strict)"("Visible"=w256) -> ()  [unwired: 2 in, 2 out]
      }
    }
    n224 = Not Equal?(x=w248, y=w245) -> (x != y?=w247:bool)
    n225 = case shown="True" w247 {
      selector: w247 -> [w262 w274]
      tunnel: w245 -> [_ w277]
      tunnel: w240 -> [_ w276]
      tunnel: [w262 w274] -> w236
      frame False {
      }
      frame True {
        n226 = local read "Sensitivity"() -> (w270:dbl)
        n227 = local read "Vp Out"() -> (w269:dbl)
        n228 = Compound Arithmetic op=MULTIPLY(w269, w270) -> (w268:dbl)
        n229 = Divide(x=w268, y=5.0 ("x")) -> (x/y=w267:dbl)
        n230 = case shown="2, 3" w277 {
          tunnel: [TRUE w328 FALSE] -> w281
          tunnel: [w319 w327 FALSE] -> w272
          tunnel: [w322 0.0 ("wav ol min") 0.0 ("wav ol min")] -> w283
          tunnel: [w321 w325 w330] -> w284
          tunnel: [w320 w329 w333] -> w285
          tunnel: [w319 w328 w334] -> w280
          tunnel: [w319 w327 w334] -> w264
          tunnel: [w318 FALSE ("Mute") FALSE ("Mute")] -> w282
          tunnel: w267 -> [_ w325 w330]
          frame 0, Default {
            w319 = FALSE
            n231 = local read "sine ol max"() -> (w321:dbl)
            n232 = local read "sine ol min"() -> (w322:dbl)
            n233 = local read "sine ol log"() -> (w320:bool)
            n234 = local read "Mute"() -> (w318:bool)
          }
          frame 1 {
            w327 = TRUE
            w328 = FALSE
            n235 = local read "wav ol log"() -> (w329:bool)
          }
          frame 2, 3 {
            w334 = TRUE
            n236 = local read "wav ol log"() -> (w333:bool)
          }
        }
        n237 = property on="Frequency" class="Knob (strict)"("Visible"=w281) -> ()  [unwired: 2 in, 2 out]
        n238 = property on="lin1" class="Bool (strict)"("Visible"=w281) -> ()  [unwired: 2 in, 2 out]
        n239 = property on="1 kHz" class="Bool"("Visible"=w281) -> ()  [unwired: 2 in, 2 out]
        n240 = property on="Output Level(RMS)" class="Knob (strict)"("Scale.Range:Minimum"=w283, "Scale.Range:Maximum"=w284) -> (error out=w273:errorcluster)  [unwired: 2 in, 1 out]
        n241 = property on="freq lin/log" class="Bool (strict)"("Visible"=w281) -> ()  [unwired: 2 in, 2 out]
        n242 = property on="Wave path" class="Str"("Visible"=w272) -> ()  [unwired: 2 in, 2 out]
        n243 = property on="Peak" class="DigNum (strict)"("Visible"=w272) -> ()  [unwired: 2 in, 2 out]
        n244 = property on="RMS" class="DigNum (strict)"("Visible"=w272) -> ()  [unwired: 2 in, 2 out]
        n245 = property on="stereo" class="Str"("Visible"=w272) -> ()  [unwired: 2 in, 2 out]
        n246 = property on="Max(Hz)" class="DigNum (strict)"("Visible"=w280) -> ()  [unwired: 2 in, 2 out]
        n247 = property on="Wave play mode" class="Slide (strict)"("Visible"=w264) -> ()  [unwired: 2 in, 2 out]
        n248 = property on="stop" class="Bool"("Visible"=w264) -> ()  [unwired: 2 in, 2 out]
        n249 = local write "level lin/log"(w285) -> ()
        n250 = local write "mute flash"(w282) -> ()
        n251 = property on="OK1" class="Bool (strict)"("Visible"=w264) -> ()  [unwired: 2 in, 2 out]
        n252 = Not(x=w264) -> (.not. x?=w263:bool)
        n253 = property on="start" class="Bool (strict)"("Visible"=w264) -> ()  [unwired: 2 in, 2 out]
        n254 = property on="Cancel" class="Bool (strict)"("Visible"=w281) -> ()  [unwired: 2 in, 2 out]
        n255 = property on="Browse" class="Bool"("Visible"=w272) -> ()  [unwired: 2 in, 2 out]
        n256 = property on="Peak Unit" class="Ring (strict)"("Visible"=w272) -> ()  [unwired: 2 in, 2 out]
        n257 = property on="RMS Unit" class="Ring (strict)"("Visible"=w272) -> ()  [unwired: 2 in, 2 out]
        n258 = property on="Time" class="Str"("Visible"=w272) -> ()  [unwired: 2 in, 2 out]
        n259 = property on="unit1" class="Str"("Visible"=w281) -> ()  [unwired: 2 in, 2 out]
        n260 = property on="log1" class="Bool (strict)"("Visible"=w281) -> ()  [unwired: 2 in, 2 out]
        n261 = property on="Min (Hz)" class="DigNum (strict)"("Visible"=w280) -> ()  [unwired: 2 in, 2 out]
        n262 = property on="Duration(s)" class="DigNum (strict)"("Visible"=w280) -> ()  [unwired: 2 in, 2 out]
        n263 = property on="cancel2" class="Bool (strict)"("Visible"=w264) -> ()  [unwired: 2 in, 2 out]
        n264 = property on="Mute" class="Bool (strict)"("Visible"=w281) -> ()  [unwired: 2 in, 2 out]
        n265 = property on="OK" class="Bool (strict)"("Visible"=w263) -> ()  [unwired: 2 in, 2 out]
        n266 = property on="Sel Channel" class="Ring (strict)"("Visible"=w272) -> ()  [unwired: 2 in, 2 out]
        n267 = case shown="True" w276 {
          tunnel: w281 -> [w316 _]
          frame False {
            n268 = property on="Play Sine Wave:" class="Slide (strict)"("Visible"=w316) -> ()  [unwired: 2 in, 2 out]
          }
          frame True {
            n269 = property on="Play Sine Wave:" class="Slide (strict)"("Visible"=FALSE) -> ()  [unwired: 2 in, 2 out]
          }
        }
        n270 = case shown="No Error" w273 {
          frame No Error {
          }
          frame Error {
          }
        }
        n271 = property on="mute border" class="Bool (strict)"("Visible"=w281) -> ()  [unwired: 2 in, 2 out]
        n272 = case shown="False" w276 {
          tunnel: w264 -> [w296 w314]
          tunnel: w264 -> [w297 w315]
          tunnel: [w295 w315] -> w278
          tunnel: [w294 w314] -> w279
          tunnel: w277 -> [w298 _]
          frame False {
            n273 = case shown="1..3" w298 {
              tunnel: w297 -> [w301 w308]
              tunnel: w296 -> [w299 w307]
              tunnel: [w301 w308] -> w295
              tunnel: [w299 w307] -> w294
              frame 0, Default {
                n274 = property on="Duration" class="DigNum (strict)"("Disabled"=u8 0) -> ()  [unwired: 2 in, 2 out]
              }
              frame 1..3 {
                n275 = local read "Wave play mode"() -> (w302:i32)
                n276 = case shown="1" w302 {
                  tunnel: [w309 w311 w312] -> w304
                  tunnel: u8 2 ("Write Attribute") -> [w309 w310 w312]
                  tunnel: [w309 w310 w313] -> w305
                  tunnel: u8 0 ("Write Attribute") -> [_ w311 w313]
                  frame 0, Default {
                  }
                  frame 1 {
                  }
                  frame 2 {
                  }
                }
                n277 = property on="Duration" class="DigNum (strict)"("Disabled"=w304) -> ()  [unwired: 2 in, 2 out]
                n278 = property on="n times" class="DigNum (strict)"("Disabled"=w305) -> ()  [unwired: 2 in, 2 out]
              }
            }
          }
          frame True {
          }
        }
        n279 = local read "asio inited"() -> (w265:bool)
        n280 = local read "Audio Driver"() -> (w266:u16)
        n281 = local write "ReMake Flg"(FALSE ("ReMake Flg")) -> ()
        n282 = case shown="2" w266 {
          tunnel: w265 -> [_ w286]
          frame 0, Default {
          }
          frame 2 {
            n283 = case shown="True" w286 {
              frame False {
              }
              frame True {
                n284 = local read "Channel Out"() -> (w290:u32)
                n285 = local read "Gen_Index"() -> (w289:i32)
                n286 = local read "isMain"() -> (w288:bool)
                n287 = local read "Asio OCI"() -> (w291:u32)
                n288 = local write "asio inited"(FALSE ("asio start")) -> ()
                n289 = call "CRYASIO Close Cur Channel & Dev.vi"("Limit"=w291, "isInput?"=FALSE, "Channel Out"=w290) -> ()  [unwired: 9 in]
                n290 = call "CRYClear Main Generator Array.vi"("isMain"=w288, "Gen Idx"=w289) -> ("isMain out"=w287:bool)  [unwired: 9 in]
                n291 = local write "isMain"(w287) -> ()
              }
            }
          }
        }
        n292 = property on="n times" class="DigNum (strict)"("Visible"=w278) -> ()  [unwired: 2 in, 2 out]
        n293 = property on="Duration" class="DigNum (strict)"("Visible"=w279) -> ()  [unwired: 2 in, 2 out]
      }
    }
    n294 = case shown="1..3" w245 {
      tunnel: [w352 w776] -> w255
      tunnel: [w356 w791] -> w249
      tunnel: [w359 w775] -> w254
      tunnel: w253 -> [w359 w768]
      tunnel: w252 -> [w349 w767]
      tunnel: [w348 w790] -> w251
      tunnel: [w360 w792] -> w250
      tunnel: w241 -> [w350 w774]
      tunnel: w239 -> [w343 _]
      tunnel: w238 -> [w347 _]
      tunnel: [w346 i16 -1 ("Channel")] -> w237
      tunnel: w236 -> [_ _]
      tunnel: [w345 0 ("Buffer Amount")] -> w235
      tunnel: w234 -> [w344 _]
      tunnel: w233 -> [w339 w760]
      tunnel: w232 -> [w338 w759]
      tunnel: w231 -> [w337 w758]
      tunnel: [w342 w760] -> w230
      tunnel: [w341 w759] -> w229
      tunnel: [w340 w758] -> w228
      frame 0, Default {
        w360 = errorcluster {"status"=FALSE, "code"=0, "source"=""}  # no error
        # "Sine Wave Play"
        n295 = while {
          shift-right: [w383] -> w342
          shift-left: w339 -> [w384]
          shift-right: [w382] -> w346
          shift-left: w347 -> [w366]
          tunnel: [w377] -> w356
          shift-right: [w380] -> w354
          shift-left: FALSE ("Quadrature") -> [w381]
          shift-right: [w378] -> _
          shift-left: FALSE ("Quadrature") -> [w379]
          tunnel: [w374] -> w352
          tunnel: w350 -> [w372]
          shift-right: [w371] -> w341
          shift-left: w338 -> [w370]
          shift-right: [w368] -> w340
          shift-left: w337 -> [w369]
          tunnel: w343 -> [w367]
          tunnel: w349 -> [_]
          shift-right: [w365] -> w345
          shift-left: w344 -> [w364]
          i -> [w363]
          stop <- w376 continue-if-true
          n296 = Equal To 0?(x=w363) -> (x = 0?=w375:bool)
          n297 = Wait Until Next ms Multiple(millisecond multiple=u32 10 ("milliseconds to wait")) -> ()  [unwired: 1 out]
          n298 = stacked-sequence {
            tunnel: [w385 _ _ _ _] -> w382
            tunnel: w366 -> [w387 _ w486 _ w580]
            tunnel: [_ _ _ _ w567] -> w376
            tunnel: [_ _ _ _ w570] -> w374
            tunnel: [_ _ _ _ w581] -> w383
            tunnel: w384 -> [_ _ _ _ w597]
            tunnel: [_ _ _ _ w577] -> w377
            tunnel: w381 -> [_ _ _ w540 _]
            tunnel: [_ _ _ w537 _] -> w380
            tunnel: w379 -> [_ _ _ w535 _]
            tunnel: [_ _ _ w533 _] -> w378
            tunnel: w375 -> [_ _ _ w532 _]
            tunnel: w372 -> [_ _ _ _ w566]
            tunnel: w367 -> [_ w464 _ _ _]
            tunnel: w370 -> [_ _ w489 _ _]
            tunnel: [_ _ w488 _ _] -> w371
            tunnel: w369 -> [_ _ w484 _ _]
            tunnel: [_ _ w483 _ _] -> w368
            tunnel: [_ _ _ _ w556] -> w365
            tunnel: w364 -> [_ _ _ _ w553]
            frame #0 {
              n299 = property on="Signal Path" class="Ring (strict)"() -> ("Value"=w385:i16)  [unwired: 2 in, 2 out]
              n300 = Not Equal?(x=w387, y=w385) -> (x != y?=w386:bool)
              n301 = case shown="True" w386 {
                frame False {
                }
                frame True {
                  n302 = flat-sequence {
                    frame #0 {
                      n303 = local read "Audio Driver"() -> (w389:u16)
                      n304 = local read "asio inited"() -> (w388:bool)
                      n305 = case shown="2" w389 {
                        tunnel: w388 -> [_ w394]
                        frame 0, Default {
                          w393 = 0.0 ("OutFrequency")
                          w392 = u32 0 ("DeviceID")
                          n306 = local read "ntaskID"() -> (w390:u32)
                          n307 = local read "Audio Driver"() -> (w391:u16)
                          n308 = dll-call lib="D:/A_CRYSoundLab_Work/CRY6181/CRYSound.dll" fn="GVPlaySine"("DeviceID"=w391, "OutSampleFreq"=w392, "nOutbitDepth"=w392, "nOutChannels"=w392, "OutFrequency"=w393, "PlayMode"=w392, "Duration"=w393, "nTimes"=w392, "OutLevel"=w393, "startflag"=w392, "pauseflag"=w392, "changeflag"=w392, "ntaskID"=w390) -> ()  [unwired: 13 in, 6 out]
                        }
                        frame 2 {
                          n309 = case shown="True" w394 {
                            frame False {
                            }
                            frame True {
                              n310 = local read "isMain"() -> (w396:bool)
                              n311 = local read "Gen_Index"() -> (w395:i32)
                              n312 = local read "Channel Out"() -> (w399:u32)
                              n313 = local read "Asio OCI"() -> (w397:u32)
                              n314 = local write "asio inited"(FALSE ("asio start")) -> ()
                              n315 = call "CRYASIO Close Cur Channel & Dev.vi"("Limit"=w397, "isInput?"=FALSE, "Channel Out"=w399) -> ()  [unwired: 9 in]
                              n316 = call "CRYClear Main Generator Array.vi"("isMain"=w396, "Gen Idx"=w395) -> ()  [unwired: 9 in, 1 out]
                            }
                          }
                        }
                      }
                    }
                    frame #1 {
                      n317 = property on="Signal Path" class="Ring (strict)"() -> ("RingText.Text"=w414:string)  [unwired: 2 in, 2 out]
                      n318 = local read "Calibration in"() -> (w412:string)
                      n319 = local read "Hardware in"() -> (w413:string)
                      n320 = call "CRYGet Current Calibration Info.vi"("Is Input?"=FALSE, "Signal Type Name"=w414) -> ("Calibration All Cluster"=w425:T7)  [unwired: 9 out]
                      n321 = call "CRYGet Hardware Info From Signal Type.vi"("Calibration In"=w412, "Hardware In"=w413, "Signal Type"=w414, "In/Out?"=FALSE) -> ("Channel Info Out"=w411:T12)  [unwired: 5 in, 2 out]
                      n322 = Unbundle By Name(w425) -> ("EQ Curve"=w443:T9, "Sens Curve"=w441:T9)
                      n323 = Unbundle By Name(w411) -> ("ID"=w438:i32, "Hardware Ch ID"=w407:u8, "Sampling Rate (Hz)"=w436:u32, "Bit Depth"=w437:u32, "Vmax (V)"=w410:dbl, "Audio Driver"=w408:u16, "Device Name"=w409:string)
                      n324 = Unbundle By Name(w441) -> ("Curve"=w439:cluster{"x":dbl, "y":dbl, "z":dbl}[], "Y unit"=w405:string, "Y dB ref"=w430:dbl)
                      n325 = Unbundle By Name(w443) -> ("Curve"=w442:cluster{"x":dbl, "y":dbl, "z":dbl}[])  [unwired: 1 out]
                      n326 = local write "Output Device"(w438) -> ()
                      n327 = local write "Audio Driver"(w408) -> ()
                      n328 = local write "Device Name"(w409) -> ()
                      n329 = local write "Channel Out"(w407) -> ()
                      n330 = local write "BitDepth"(w437) -> ()
                      n331 = local write "Fs"(w436) -> ()
                      n332 = local write "Equalization Out"(w442) -> ()
                      n333 = Reverse String(1:w405) -> (0:w403:string)
                      n334 = Index Array(array=w439) -> (element=w440:cluster{"x":dbl, "y":dbl, "z":dbl})  [unwired: 1 in]
                      n335 = Unbundle By Name(w440) -> ("y"=w433:dbl)
                      n336 = Match Pattern(string=w403, regular expression="/" ("search char (-)")) -> (after substring=w401:string)  [unwired: 1 in, 3 out]
                      n337 = Less Or Equal To 0?(x=w433) -> (x <= 0?=w435:bool)
                      n338 = Reverse String(1:w401) -> (0:w404:string)
                      n339 = case shown="2" w408 {
                        tunnel: w407 -> [_ w448]
                        frame 0, Default {
                          n340 = local read "Gen_Index"() -> (w446:i32)
                          n341 = call "CRYUpdate Generator Index.vi"("Chn Idx"=-1, "Gen_Index"=w446) -> ()  [unwired: 9 in]
                        }
                        frame 2 {
                          n342 = local read "Gen_Index"() -> (w447:i32)
                          n343 = call "CRYUpdate Generator Index.vi"("Chn Idx"=w448, "Gen_Index"=w447) -> ()  [unwired: 9 in]
                        }
                      }
                      n344 = Select(t=1.0 ("Sensitivity"), s=w435, f=w433) -> (s? t:f=w428:dbl)
                      n345 = local write "unit2"(w404) -> ()
                      n346 = global read "CRYCal Global.vi" "Calibrate"() -> (w429:bool)
                      n347 = Less Or Equal To 0?(x=w430) -> (x <= 0?=w431:bool)
                      n348 = Select(t=1.0 ("Sensitivity"), s=w431, f=w430) -> (s? t:f=w427:dbl)
                      n349 = case shown="True" w429 {
                        tunnel: w428 -> [w450 _]
                        tunnel: [w450 w451] -> w416
                        tunnel: w427 -> [w449 _]
                        tunnel: [w449 1.0 ("y")] -> w426
                        frame False {
                        }
                        frame True {
                          n350 = global read "CRYCal Global.vi" "Sens Out"() -> (w451:dbl)
                        }
                      }
                      n351 = local write "Sensitivity"(w416) -> ()
                      n352 = local write "dB ref."(w426) -> ()
                      n353 = Square Root(x=2.0) -> (sqrt(x)=w421:dbl)
                      n354 = Multiply(x=w410, y=w421) -> (x*y=w420:dbl)
                      n355 = local write "Vp Out"(w410) -> ()
                      n356 = Divide(x=w420, y=2.0) -> (x/y=w424:dbl)
                      n357 = Multiply(x=w424, y=w416) -> (x*y=w417:dbl)
                      n358 = property on="Output Level(RMS)" class="Knob (strict)"("Maximum"=w417, "Scale.Maximum"=w417, "Scale.Minimum"=0.0 ("Scale.Range:Minimum")) -> (error out=w418:errorcluster)  [unwired: 2 in, 1 out]
                      n359 = local write "isMain"(FALSE ("isMain")) -> ()
                      n360 = case shown="No Error" w418 {
                        frame No Error {
                        }
                        frame Error {
                        }
                      }
                    }
                    frame #2 {
                      n361 = local read "asio inited"() -> (w453:bool)
                      n362 = local read "Audio Driver"() -> (w454:u16)
                      n363 = case shown="2" w454 {
                        tunnel: w453 -> [_ w455]
                        frame 0, Default {
                        }
                        frame 2 {
                          n364 = case shown="False" w455 {
                            frame False {
                              n365 = local read "Channel Out"() -> (w461:u32)
                              n366 = local read "BitDepth"() -> (w459:u32)
                              n367 = local read "Gen_Index"() -> (w458:i32)
                              n368 = local read "Fs"() -> (w460:u32)
                              n369 = local read "Device Name"() -> (w463:string)
                              n370 = call "CRYASIO Out & Init & Start.vi"("Bit Depth"=w459, "Sampling Rate"=w460, "Channel Index"=w461, "Device Name"=w463) -> ("bResult"=w456:bool, "Asio Opend Channel Index"=w462:u32)  [unwired: 6 in]
                              n371 = local write "asio inited"(w456) -> ()
                              n372 = local write "Asio OCI"(w462) -> ()
                              n373 = call "CRYSet Main Generator Array.vi"("Gen Idx"=w458) -> ("Is Main?"=w457:bool)  [unwired: 10 in]
                              n374 = local write "isMain"(w457) -> ()
                            }
                            frame True {
                            }
                          }
                        }
                      }
                    }
                  }
                }
              }
            }
            frame #1 {
              n375 = case shown="True" "1 kHz" {
                frame False {
                }
                frame True {
                  n376 = local write "Frequency"(1000.0 ("Frequency")) -> ()
                }
              }
              n377 = local read "Mute"() -> (w465:bool)
              n378 = case shown="True" w465 {
                selector: w465 -> [w467 _]
                tunnel: w464 -> [_ w468]
                frame False {
                  n379 = local write "mute border"(w467) -> ()
                }
                frame True {
                  n380 = Quotient & Remainder(x=w468, y=70) -> (x-y*floor(x/y)=w474:i32)  [unwired: 1 out]
                  n381 = Equal To 0?(x=w474) -> (x = 0?=w469:bool)
                  n382 = local read "mute border"() -> (w472:bool)
                  n383 = local read "Mute"() -> (w470:bool)
                  n384 = Compound Arithmetic op=AND(w470, w469) -> (w471:bool)
                  n385 = case shown="True" w471 {
                    tunnel: w472 -> [_ w477]
                    frame False {
                      n386 = Wait (ms)(milliseconds to wait=u32 10) -> ()  [unwired: 1 out]
                    }
                    frame True {
                      n387 = Not(x=w477) -> (.not. x?=w476:bool)
                      n388 = local write "mute border"(w476) -> ()
                    }
                  }
                }
              }
            }
            frame #2 {
              n389 = local read "Output Level(RMS)"() -> (w491:dbl)
              n390 = local read "Signal Path"() -> (w487:i16)
              n391 = local read "dB"() -> (w481:dbl)
              n392 = Not Equal?(x=w481, y=w484) -> (x != y?=w479:bool)
              n393 = Not Equal?(x=w489, y=w491) -> (x != y?=w490:bool)
              n394 = Not Equal?(x=w486, y=w487) -> (x != y?=w485:bool)
              n395 = Or(x=w490, y=w485) -> (x .or. y?=w482:bool)
              n396 = Or(x=w482, y=w479) -> (x .or. y?=w480:bool)
              n397 = case shown="True" w480 {
                tunnel: w491 -> [w493 w499]
                tunnel: [w493 w498] -> w488
                tunnel: w484 -> [w492 _]
                tunnel: [w492 w497] -> w483
                tunnel: w482 -> [_ w494]
                tunnel: w481 -> [_ w496]
                tunnel: w479 -> [_ w495]
                frame False {
                }
                frame True {
                  n398 = case shown="False" w494 {
                    tunnel: w499 -> [_ w531]
                    tunnel: [w500 w517] -> w498
                    tunnel: [w502 w516] -> w497
                    tunnel: w496 -> [w501 _]
                    tunnel: w495 -> [_ _]
                    frame False {
                      n399 = local read "dB ref."() -> (w503:dbl)
                      n400 = call "CRYConversion dB-Lin.vi"("dB ref."=w503, "Log In"=w501) -> ("Lin Out"=w505:dbl)  [unwired: 4 in, 3 out]
                      n401 = property on="Output Level(RMS)" class="Knob (strict)"() -> ("Maximum"=w506:dbl)  [unwired: 2 in, 2 out]
                      n402 = Greater?(x=w505, y=w506) -> (0:w504:bool)
                      n403 = case shown="True" w504 {
                        tunnel: w506 -> [_ w510]
                        tunnel: [w508 w509] -> w502
                        tunnel: w501 -> [w508 _]
                        tunnel: w505 -> [w507 _]
                        tunnel: [w507 w510] -> w500
                        frame False {
                        }
                        frame True {
                          n404 = local read "dB ref."() -> (w514:dbl)
                          n405 = Less?(x=w510, y=1e-05) -> (x < y?=w512:bool)
                          n406 = call "CRYConversion dB-Lin.vi"("dB ref."=w514, "Lin In"=w510) -> ("Log Out"=w515:dbl)  [unwired: 4 in, 3 out]
                          n407 = Select(t=-1000.0, s=w512, f=w515) -> (s? t:f=w509:dbl)
                          n408 = local write "dB"(w509) -> ()
                        }
                      }
                      n409 = local write "sine level"(w500) -> ()
                      n410 = local write "Output Level(RMS)"(w500) -> ()
                    }
                    frame True {
                      n411 = local read "Vp Out"() -> (w524:dbl)
                      n412 = Square Root(x=2.0) -> (sqrt(x)=w527:dbl)
                      n413 = local read "Sensitivity"() -> (w529:dbl)
                      n414 = Multiply(x=w524, y=w527) -> (x*y=w528:dbl)
                      n415 = Divide(x=w528, y=2.0) -> (x/y=w523:dbl)
                      n416 = Multiply(x=w523, y=w529) -> (x*y=w530:dbl)
                      n417 = Max & Min(x=w531, y=w530) -> (min(x,y)=w517:dbl)  [unwired: 1 out]
                      n418 = local read "dB ref."() -> (w521:dbl)
                      n419 = Less?(x=w517, y=1e-05) -> (x < y?=w519:bool)
                      n420 = call "CRYConversion dB-Lin.vi"("dB ref."=w521, "Lin In"=w517) -> ("Log Out"=w522:dbl)  [unwired: 4 in, 3 out]
                      n421 = Select(t=-1000.0, s=w519, f=w522) -> (s? t:f=w516:dbl)
                      n422 = local write "sine level"(w517) -> ()
                      n423 = local write "Output Level(RMS)"(w517) -> ()
                      n424 = local write "dB"(w516) -> ()
                    }
                  }
                }
              }
            }
            frame #3 {
              n425 = local read "level lin/log"() -> (w537:bool)
              n426 = local read "freq lin/log"() -> (w533:bool)
              n427 = Exclusive Or(1:w533, 2:w535) -> (0:w536:bool)
              n428 = Exclusive Or(1:w537, 2:w540) -> (0:w539:bool)
              n429 = Or(x=w539, y=w532) -> (x .or. y?=w538:bool)
              n430 = Or(x=w536, y=w532) -> (x .or. y?=w534:bool)
              n431 = case shown="True" w538 {
                tunnel: w537 -> [w545 _]
                frame True {
                  n432 = Select(t=u8 1 ("Write Attribute"), s=w545, f=u8 0 ("Write Attribute")) -> (s? t:f=w548:u8)
                  n433 = property on="Output Level(RMS)" class="Knob (strict)"("Scale.Mapping Mode"=w548) -> ()  [unwired: 2 in, 2 out]
                }
                frame False {
                }
              }
              n434 = case shown="True" w534 {
                tunnel: w533 -> [_ w541]
                frame False {
                }
                frame True {
                  n435 = Select(t=u8 1 ("Write Attribute"), s=w541, f=u8 0 ("Write Attribute")) -> (s? t:f=w544:u8)
                  n436 = property on="Frequency" class="Knob (strict)"("Scale.Mapping Mode"=w544) -> ()  [unwired: 2 in, 2 out]
                }
              }
            }
            frame #4 {
              w582 = 0.0
              n437 = property on="Signal Path" class="Ring (strict)"() -> ("Value"=w554:i16)  [unwired: 2 in, 2 out]
              n438 = local read "EQ"() -> (w573:bool)
              n439 = local read "Output Level(RMS)"() -> (w591:dbl)
              n440 = local read "OK"() -> (w549:bool)
              n441 = global read "CRYMainGlobal.vi" "Acq Stop"() -> (w564:bool)
              n442 = global read "CRYProject Run Control Global.vi" "Cont Seq"() -> (w560:bool)
              n443 = global read "CRYProject Run Control Global.vi" "Aborted"() -> (w562:bool)
              n444 = global read "CRYMainGlobal.vi" "STOP"() -> (w572:bool)
              n445 = local read "Vp Out"() -> (w592:dbl)
              n446 = local read "Signal Type"() -> (w565:i32)
              n447 = Square Root(x=2.0) -> (sqrt(x)=w588:dbl)
              n448 = local read "Mute"() -> (w586:bool)
              n449 = Max & Min(x=w591, y=w582) -> (max(x,y)=w593:dbl)  [unwired: 1 out]
              n450 = Divide(x=w588, y=w592) -> (x/y=w595:dbl)
              n451 = Compound Arithmetic op=OR(w549, "Cancel", w572, w564, w562, w560) -> (w570:bool)
              n452 = local read "Frequency"() -> (w581:dbl)
              n453 = case shown="True" w573 {
                tunnel: w581 -> [_ w744]
                tunnel: [1.0 w743] -> w579
                frame False {
                }
                frame True {
                  n454 = local read "Equalization Out"() -> (w748:cluster{"Hz":dbl, dbl, "Deg":dbl}[])
                  n455 = Sort 1D Array(array=w748) -> (sorted array=w747:cluster{"Hz":dbl, dbl, "Deg":dbl}[])
                  n456 = for {
                    tunnel: w747 -> [w753] mode=indexing
                    tunnel: [w749] -> w746 mode=indexing
                    n457 = Unbundle(w753) -> ("Hz"=w752:dbl, w750:dbl)  [unwired: 1 out]
                    n458 = Logarithm Base 10(1:w752) -> (0:w751:dbl)
                    n459 = Bundle(w751, w750) -> (w749:cluster{dbl, dbl})  [unwired: 1 out]
                  }
                  n460 = Logarithm Base 10(1:w744) -> (0:w745:dbl)
                  n461 = Interpolate 1D Array(1:w745, 2:w746) -> (0:w743:dbl)
                }
              }
              n462 = local read "Sensitivity"() -> (w590:dbl)
              n463 = Select(t=w582, s=w586, f=w593) -> (s? t:f=w589:dbl)
              n464 = local read "Play Sine Wave:"() -> (w563:i32)
              n465 = Equal To 0?(x=w565) -> (x = 0?=w578:bool)
              n466 = Not(x=w586) -> (.not. x?=w561:bool)
              n467 = local read "Output Device"() -> (w575:u32)
              n468 = local read "Audio Driver"() -> (w558:u16)
              n469 = local read "Channel Out"() -> (w569:u32)
              n470 = Not(x=w570) -> (.not. x?=w577:bool)
              n471 = Multiply(x=w589, y=w595) -> (x*y=w587:dbl)
              n472 = local read "Duration"() -> (w552:dbl)
              n473 = local read "BitDepth"() -> (w574:u32)
              n474 = Divide(x=w587, y=w590) -> (x/y=w551:dbl)
              n475 = Not Equal?(x=w554, y=w580) -> (x != y?=w555:bool)
              n476 = local read "Fs"() -> (w576:u32)
              n477 = Not Equal?(x=w581, y=w597) -> (x != y?=w585:bool)
              n478 = Compound Arithmetic op=AND(w561, w578, w577) -> (w567:bool)
              n479 = Compound Arithmetic op=OR(w555, w585) -> (w557:bool)
              n480 = Multiply(x=w551, y=w579) -> (x*y=w594:dbl)
              n481 = Boolean To (0,1)(Boolean=w557) -> (0, 1=w559:i16)
              n482 = Boolean To (0,1)(Boolean=w567) -> (0, 1=w583:i16)
              n483 = case shown="2" w558 {
                tunnel: w594 -> [w601 w740]
                tunnel: "ntaskID" -> [_ w738]
                tunnel: w583 -> [_ w734]
                tunnel: w581 -> [w619 w732]
                tunnel: w576 -> [w615 w731]
                tunnel: w575 -> [_ w730]
                tunnel: w574 -> [_ w729]
                tunnel: w569 -> [w614 w728]
                tunnel: w552 -> [_ w727]
                tunnel: w563 -> [_ w726]
                tunnel: w559 -> [_ w725]
                tunnel: [w610 w722] -> w550
                tunnel: [w618 _] -> w556
                tunnel: w553 -> [w617 _]
                tunnel: w555 -> [_ _]
                frame 2 {
                  n484 = local read "Mute"() -> (w600:bool)
                  n485 = case shown="True" w600 {
                    tunnel: [w621 w622] -> w602
                    frame False {
                      n486 = local read "Gen_Index"() -> (w620:i32)
                      n487 = call "CRYCheck Main Generator.vi"("Gen Idx"=w620) -> ("Is Main?"=w621:bool)  [unwired: 10 in]
                      n488 = local write "isMain"(w621) -> ()
                    }
                    frame True {
                      n489 = local read "Gen_Index"() -> (w624:i32)
                      n490 = local read "isMain"() -> (w623:bool)
                      n491 = call "CRYClear Main Generator Array.vi"("isMain"=w623, "Gen Idx"=w624) -> ("isMain out"=w622:bool)  [unwired: 9 in]
                      n492 = local write "isMain"(w622) -> ()
                    }
                  }
                  n493 = Less?(x=w617, y=30000) -> (x < y?=w613:bool)
                  n494 = Not(x=w600) -> (.not. x?=w612:bool)
                  n495 = local read "asio inited"() -> (w603:bool)
                  n496 = case shown="True" w603 {
                    tunnel: w619 -> [_ w633]
                    tunnel: w601 -> [_ w632]
                    tunnel: [0 ("Buffer Amount") w631] -> w618
                    tunnel: w615 -> [_ w630]
                    tunnel: w614 -> [_ w629]
                    tunnel: w613 -> [_ w628]
                    tunnel: w612 -> [_ w627]
                    tunnel: w602 -> [_ w626]
                    frame False {
                    }
                    frame True {
                      n497 = case shown="False" w626 {
                        tunnel: w633 -> [w641 w695]
                        tunnel: w632 -> [w640 w694]
                        tunnel: [w639 w693] -> w631
                        tunnel: w630 -> [w638 w692]
                        tunnel: w628 -> [w635 w691]
                        tunnel: w626 -> [w637 w690]
                        tunnel: w629 -> [w636 w689]
                        tunnel: w627 -> [w634 w688]
                        frame True {
                          n498 = case shown="True" w635 {
                            tunnel: w641 -> [w649 _]
                            tunnel: w640 -> [w648 _]
                            tunnel: [w647 w687] -> w639
                            tunnel: w638 -> [w646 _]
                            tunnel: w634 -> [w642 _]
                            tunnel: [w645 w686] -> _
                            tunnel: w637 -> [w644 _]
                            tunnel: w636 -> [w643 _]
                            frame True {
                              n499 = case shown="True" w642 {
                                tunnel: w649 -> [_ w680]
                                tunnel: w648 -> [_ w665]
                                tunnel: w646 -> [_ w679]
                                tunnel: [w654 w678] -> w647
                                tunnel: [w653 w676] -> w645
                                tunnel: w644 -> [_ _]
                                tunnel: w643 -> [w652 w673]
                                frame False {
                                n500 = call "CRYGet Global Buffer.vi"("Chn Idx"=w652) -> ("Global Buffer Out"=w650:sgl[], "isEmpty"=w651:bool)  [unwired: 8 in]
                                n501 = case shown="False" w651 {
                                tunnel: [w657 w664] -> w654
                                tunnel: [w655 w662] -> w653
                                tunnel: w650 -> [_ w660]
                                frame True {
                                n502 = local read "Asio OCI"() -> (w656:u32)
                                n503 = call "CRYASIOAddPlayBuffer.vi"("Limit"=w656, "Data Length"=0, "pData"=sgl[] []) -> ("Buffer Amount"=w657:i32, "bResult"=w655:bool)  [unwired: 5 in, 1 out]
                                }
                                frame False {
                                n504 = local read "Asio OCI"() -> (w663:u32)
                                n505 = Array Size(array=w660) -> (size(s)=w661:i32)
                                n506 = call "CRYASIOAddPlayBuffer.vi"("Limit"=w663, "Data Length"=w661, "pData"=w660) -> ("Buffer Amount"=w664:i32, "bResult"=w662:bool)  [unwired: 5 in, 1 out]
                                }
                                }
                                }
                                frame True {
                                w674 = 2048 ("# of samples")
                                n507 = Divide(x=w674, y=w679) -> (x/y=w668:dbl)
                                n508 = local read "Dur_asio"() -> (w669:dbl)
                                n509 = call <vilib>:"Signal Generator by Duration.vi"("signal type"=T13."sine", "duration"=w668, "reset phase"=FALSE, "# of samples"=w674, "frequency"=w680, "amplitude"=w665) -> ("signal"=w666:dbl[])  [unwired: 6 in, 3 out]
                                n510 = Subtract(x=w669, y=w668) -> (x-y=w667:dbl)
                                n511 = To Single Precision Float(number=w666) -> (single precision float=w672:sgl[])
                                n512 = local write "Dur_asio"(w667) -> ()
                                n513 = call "CRYGet Global Buffer.vi"("Chn Idx"=w673) -> ("Global Buffer Out"=w671:sgl[])  [unwired: 8 in, 1 out]
                                n514 = Add(x=w672, y=w671) -> (x+y=w670:sgl[])
                                n515 = Array Size(array=w670) -> (size(s)=w681:i32)
                                n516 = local read "Asio OCI"() -> (w677:u32)
                                n517 = call "CRYASIOAddPlayBuffer.vi"("Limit"=w677, "Data Length"=w681, "pData"=w670) -> ("Buffer Amount"=w678:i32, "bResult"=w676:bool)  [unwired: 5 in, 1 out]
                                }
                              }
                            }
                            frame False {
                              n518 = local read "Asio OCI"() -> (w683:u32)
                              n519 = call "CRYASIOAddPlayBuffer.vi"("Limit"=w683, "Data Length"=0, "pData"=sgl[] []) -> ("Buffer Amount"=w687:i32, "bResult"=w686:bool)  [unwired: 5 in, 1 out]
                            }
                          }
                        }
                        frame False {
                          n520 = case shown="True" w691 {
                            tunnel: w695 -> [_ w719]
                            tunnel: w694 -> [_ w713]
                            tunnel: w692 -> [_ w718]
                            tunnel: [w697 w717] -> w693
                            tunnel: w690 -> [_ _]
                            tunnel: w689 -> [_ _]
                            tunnel: w688 -> [_ w710]
                            frame False {
                              n521 = local read "Asio OCI"() -> (w696:u32)
                              n522 = call "CRYASIOAddPlayBuffer.vi"("Limit"=w696, "Data Length"=0, "pData"=sgl[] []) -> ("Buffer Amount"=w697:i32)  [unwired: 5 in, 2 out]
                            }
                            frame True {
                              w714 = 2048 ("# of samples")
                              n523 = Divide(x=w714, y=w718) -> (x/y=w702:dbl)
                              n524 = local read "Dur_asio"() -> (w703:dbl)
                              n525 = call <vilib>:"Signal Generator by Duration.vi"("signal type"=T13."sine", "duration"=w702, "reset phase"=FALSE, "# of samples"=w714, "frequency"=w719, "amplitude"=w713) -> ("signal"=w700:dbl[])  [unwired: 6 in, 3 out]
                              n526 = Initialize Array(sgl 0.0 ("Data Length"), 2048 ("Data Length")) -> (w706:sgl[])
                              n527 = To Single Precision Float(number=w700) -> (single precision float=w709:sgl[])
                              n528 = local read "Gen_Index"() -> (w704:i32)
                              n529 = Subtract(x=w703, y=w702) -> (x-y=w701:dbl)
                              n530 = local write "Dur_asio"(w701) -> ()
                              n531 = Select(t=w709, s=w710, f=w706) -> (s? t:f=w705:sgl[])
                              n532 = call "CRYAdd Global Buffer.vi"("Gen Idx"=w704, "Data"=w705) -> ()  [unwired: 10 in]
                              n533 = local read "Asio OCI"() -> (w716:u32)
                              n534 = call "CRYASIOAddPlayBuffer.vi"("Limit"=w716, "Data Length"=0, "pData"=sgl[] []) -> ("Buffer Amount"=w717:i32)  [unwired: 5 in, 2 out]
                            }
                          }
                        }
                      }
                    }
                  }
                  "Buffer Amount" <- w618
                  n535 = local read "Dur_asio"() -> (w611:dbl)
                  n536 = local read "Play Sine Wave:"() -> (w609:i32)
                  n537 = Less Or Equal To 0?(x=w611) -> (x <= 0?=w608:bool)
                  n538 = Not Equal To 0?(x=w609) -> (x != 0?=w607:bool)
                  n539 = And(x=w608, y=w607) -> (x .and. y?=w606:bool)
                  n540 = Select(t=TRUE, s=w606, f=FALSE) -> (s? t:f=w610:bool)
                }
                frame 0, Default {
                  n541 = To Unsigned Long Integer(number=w730) -> (unsigned 32bit integer=w737:u32)
                  n542 = To Unsigned Long Integer(number=w729) -> (unsigned 32bit integer=w736:u32)
                  n543 = To Unsigned Long Integer(number=w728) -> (unsigned 32bit integer=w735:u32)
                  n544 = dll-call lib="D:/A_CRYSoundLab_Work/CRY6181/CRYSound.dll" fn="GVPlaySine"("DeviceID"=w737, "OutSampleFreq"=w731, "nOutbitDepth"=w736, "nOutChannels"=w735, "OutFrequency"=w732, "PlayMode"=w726, "Duration"=w727, "nTimes"=0, "OutLevel"=w740, "startflag"=w734, "pauseflag"=u8 0, "changeflag"=w725, "ntaskID"=w738) -> ("return type"=w723:u32, "ntaskID"=w721:u32)  [unwired: 13 in, 4 out]
                  n545 = local write "ntaskID"(w721) -> ()
                  n546 = Not Equal?(x=w723, y=u32 0) -> (x != y?=w722:bool)
                  "Out level" <- w740
                }
              }
              n547 = Compound Arithmetic op=AND(w561, w550, w566) -> (w568:bool)
              n548 = case shown="True" w568 {
                frame False {
                }
                frame True {
                  n549 = local write "Cancel"(TRUE ("cancel2")) -> ()
                }
              }
              n550 = case shown="True" w550 {
                frame False {
                }
                frame True {
                  n551 = local read "Duration"() -> (w598:dbl)
                  n552 = local write "Mute"(TRUE ("cancel2")) -> ()
                  n553 = local write "Dur_asio"(w598) -> ()
                }
              }
            }
          }
        }
        n554 = local write "sine ol log"(w354) -> ()
        n555 = stacked-sequence {
          frame #0 {
            n556 = property on="Output Level(RMS)" class="Knob (strict)"() -> ("Scale.Range:Minimum"=w362:dbl, "Scale.Range:Maximum"=w361:dbl)  [unwired: 2 in, 2 out]
            n557 = local write "sine ol max"(w361) -> ()
            n558 = local write "sine ol min"(w362) -> ()
          }
        }
        n559 = local read "Signal Path"() -> (w351:i16)
        n560 = Bundle By Name(cluster=w349, "wav init"=TRUE, "called"=FALSE, "Hardware"=w351) -> (w348:T5)
      }
      frame 1..3 {
        n561 = local read "Output Level(RMS)"() -> (w766:dbl)
        n562 = local read "Wave play mode"() -> (w788:i32)
        n563 = local read "level lin/log"() -> (w789:bool)
        n564 = local read "Wave path"() -> (w787:string)
        n565 = global read "CRYProject Run Control Global.vi" "Cont Seq"() -> (w771:bool)
        n566 = global read "CRYMainGlobal.vi" "Acq Stop"() -> (w773:bool)
        n567 = Unbundle By Name(w768) -> ("start"=w780:bool)
        n568 = local read "Peak Unit"() -> (w785:u16)
        n569 = local read "RMS Unit"() -> (w784:u16)
        n570 = global read "CRYProject Run Control Global.vi" "Aborted"() -> (w772:bool)
        n571 = local read "Cancel"() -> (w770:bool)
        n572 = global read "CRYMainGlobal.vi" "STOP"() -> (w777:bool)
        n573 = local read "dB"() -> (w761:dbl)
        n574 = Compound Arithmetic op=OR("cancel2", w777, w773, w772, w771, w770) -> (w776:bool)
        n575 = Bundle("Wave play mode"=w788, "start"="start", "Output Level(RMS)"=w766, "dB"=w761, "level lin/log"=w789) -> (w793:T14)  [unwired: 1 out]
        n576 = Or(x="OK1", y="OK") -> (x .or. y?=w754:bool)
        n577 = while {
          tunnel: w793 -> [w1185]
          tunnel: [w1182] -> w775
          tunnel: w768 -> [w1181]
          tunnel: w788 -> [w1180]
          tunnel: "start" -> [w1169]
          shift-right: [w1178] -> w781
          shift-left: w767 -> [w1179]
          tunnel: "stop" -> [w1170]
          tunnel: w754 -> [w1177]
          tunnel: w776 -> [w1176]
          tunnel: w789 -> [w1175]
          tunnel: w766 -> [w1174]
          tunnel: "Browse" -> [w1173]
          tunnel: w785 -> [w1172]
          tunnel: w784 -> [w1171]
          tunnel: w761 -> [w1168]
          i -> [w1186]
          stop <- w1184 continue-if-true
          n578 = case shown="5" w1186 {
            tunnel: w1185 -> [w1192 w1260 w1286 w1327 w1360 w1392 w1467 w1482 w1503 w1576]
            tunnel: w1173 -> [_ _ _ _ _ w1388 _ _ _ _]
            tunnel: [w1187 w1266 w1283 FALSE ("browse") FALSE w1388 FALSE FALSE ("browse") FALSE TRUE] -> w1183
            tunnel: [w1193 w1265 w1285 w1323 w1358 w1392 w1467 w1482 w1503 w1576] -> w1182
            tunnel: w1181 -> [w1196 w1270 w1284 w1326 w1365 _ _ w1483 _ _]
            tunnel: w1180 -> [_ _ _ _ _ _ _ w1479 _ _]
            tunnel: w1169 -> [w1191 w1259 _ _ _ _ _ _ _ _]
            tunnel: w1179 -> [w1195 w1263 w1288 w1328 w1362 w1386 w1468 w1481 w1505 w1575]
            tunnel: [w1194 w1262 w1287 w1324 w1362 w1385 w1468 w1480 w1504 w1575] -> w1178
            tunnel: w1170 -> [_ w1267 _ _ _ _ _ _ _ _]
            tunnel: w1177 -> [_ w1261 _ _ _ _ _ _ _ _]
            tunnel: w1176 -> [_ w1264 _ _ _ _ _ _ _ _]
            tunnel: w1175 -> [_ _ _ _ w1363 _ _ _ _ _]
            tunnel: w1174 -> [_ _ w1289 _ w1359 _ _ _ _ _]
            tunnel: w1172 -> [_ _ _ _ _ w1391 w1465 _ _ _]
            tunnel: w1171 -> [_ _ _ _ _ w1390 w1466 _ _ _]
            tunnel: w1168 -> [_ _ _ w1325 _ _ _ _ _ _]
            frame 0 {
              n579 = local read "ReMake Flg"() -> (w1189:bool)
              n580 = Unbundle By Name(w1196) -> ("start"=w1190:bool)
              n581 = Not(x=w1189) -> (.not. x?=w1188:bool)
              n582 = Compound Arithmetic op=AND(invert w1190, w1191) -> (w1187:bool)
              n583 = Or(x=w1187, y=w1188) -> ()  [unwired: 1 out]
              n584 = case shown="True" w1187 {
                tunnel: w1195 -> [w1199 w1205]
                tunnel: [w1199 w1204] -> w1194
                tunnel: w1192 -> [w1198 w1203]
                tunnel: [w1198 w1202] -> w1193
                frame False {
                  n585 = local write "asio start"(FALSE ("asio start")) -> ()
                }
                frame True {
                  w1200 = u8 2 ("Write Attribute")
                  n586 = local read "Signal Type"() -> (w1207:i32)
                  n587 = property on="Signal Path" class="Ring (strict)"("DisabledEnum"=w1200) -> ()  [unwired: 2 in, 2 out]
                  n588 = property on="Signal Type" class="Ring (strict)"("Disabled"=w1200) -> ()  [unwired: 2 in, 2 out]
                  n589 = property on="Sel Channel" class="Ring (strict)"("Disabled"=w1200) -> ()  [unwired: 2 in, 2 out]
                  n590 = local write "asio start"(TRUE ("asio start")) -> ()
                  n591 = case shown="2, 3" w1207 {
                    selector: w1207 -> [_ w1228]
                    tunnel: [errorcluster {"status"=FALSE, "code"=0, "source"=""} ("error out") w1227] -> w1206
                    frame 0, Default {
                    }
                    frame 2, 3 {
                      # "noise"
                      n592 = disable-structure shown="Enabled" {
                        disable-tunnel: [w1229 FALSE ("ReMake Flg")] -> w1226
                        frame Disabled {
                          n593 = local read "ReMake Flg"() -> (w1229:bool)
                        }
                        frame Enabled {
                        }
                      }
                      n594 = case shown="False" w1226 {
                        tunnel: w1228 -> [w1252 _]
                        tunnel: [w1247 errorcluster {"status"=FALSE, "code"=0, "source"=""} ("error out")] -> w1227
                        frame False {
                          n595 = local read "Sensitivity"() -> (w1240:dbl)
                          n596 = local read "Vp Out"() -> (w1232:dbl)
                          n597 = local read "Output Level(RMS)"() -> (w1234:dbl)
                          n598 = case shown="2" w1252 {
                            tunnel: [w1256 w1257] -> w1251
                            frame 3, Default {
                              w1256 = u16 0 items=["White Noise", "Pink Noise"] ("Noise type")
                            }
                            frame 2 {
                              w1257 = u16 1 items=["White Noise", "Pink Noise"] ("Noise type")
                            }
                          }
                          n599 = local read "Duration(s)"() -> (w1253:dbl)
                          n600 = local read "Min (Hz)"() -> (w1255:dbl)
                          n601 = local read "Max(Hz)"() -> (w1254:dbl)
                          n602 = Multiply(x=w1232, y=w1240) -> (x*y=w1237:dbl)
                          n603 = Divide(x=w1237, y=5.0) -> (x/y=w1235:dbl)
                          n604 = local read "Fs"() -> (w1250:u32)
                          n605 = Bundle("Level Type"=u16 0, "Vp Out"=w1232, "Output Level(RMS)"=1.0) -> (w1241:T15)  [unwired: 1 in]
                          n606 = call "CRYNoise White Pink.vi"("Fs"=w1250, "Setting Infor"=w1241, "Min Frequency"=w1255, "Max Frequency"=w1254, "Time(s)"=w1253, "Amplitude"=w1234, "Noise type"=w1251) -> ("Noise"=→"noise" →"Play noise":sgl[], "sample size"=w1245:u32, "error out"=w1247:errorcluster)  [unwired: 3 in, 3 out]
                          n607 = Multiply(x=w1245, y=u32 4) -> (x*y=→"Byte num":u32)
                          n608 = Greater?(x=w1234, y=w1235) -> (0:w1236:bool)
                          n609 = Select(t=w1235, s=w1236, f=w1234) -> (s? t:f=w1233:dbl)
                          n610 = local write "Output Level(RMS)"(w1233) -> ()
                          n611 = local write "wav level"(w1233) -> ()
                          n612 = property on="Output Level(RMS)" class="Knob (strict)"("Maximum"=w1235, "Scale.Maximum"=w1235, "Scale.Minimum"=0.0 ("Scale.Range:Minimum")) -> (error out=w1243:errorcluster)  [unwired: 2 in, 1 out]
                          n613 = local write "ReMake Flg"(TRUE ("ReMake Flg")) -> ()
                          n614 = case shown="No Error" w1243 {
                            frame No Error {
                            }
                            frame Error {
                            }
                          }
                        }
                        frame True {
                        }
                      }
                    }
                  }
                  n615 = case shown="No Error" w1206 {
                    tunnel: [w1211 w1218] -> w1204
                    tunnel: w1205 -> [w1210 w1219]
                    tunnel: w1203 -> [w1209 w1222]
                    tunnel: [w1208 w1221] -> w1202
                    frame No Error {
                      w1212 = TRUE ("Bundle Element")
                      w1213 = FALSE ("Bundle Element")
                      n616 = Bundle By Name(cluster=w1210, "halt now"=w1213, "dll done"=w1213) -> (w1211:T5)
                      n617 = local write "start"(w1212) -> ()
                      n618 = Bundle By Name(cluster=w1209, "start"=w1212) -> (w1208:T14)
                    }
                    frame Error {
                      w1220 = TRUE ("Bundle Element")
                      n619 = Bundle By Name(cluster=w1219, "halt now"=w1220, "dll done"=w1220) -> (w1218:T5)
                      n620 = local write "start"(FALSE ("start")) -> ()
                      n621 = Bundle By Name(cluster=w1222, "start"=FALSE) -> (w1221:T14)
                      n622 = call "CRYGet Error Message.vi"("Error No"=0, "Kind"="Signal Generator") -> ("Message"=w1214:string, "Window Title"=w1215:string)  [unwired: 4 in, 4 out]
                      n623 = call "CRYMessage Dialog.vi"("Window Title"=w1215, "Message Content"=w1214) -> ()  [unwired: 8 in, 2 out]
                    }
                  }
                }
              }
            }
            frame 1 {
              n624 = Unbundle By Name(w1270) -> ("start"=w1269:bool)
              n625 = Compound Arithmetic op=AND(w1269, invert w1259) -> (w1268:bool)
              n626 = Compound Arithmetic op=OR(w1268, w1267, w1261, w1264) -> (w1266:bool)
              n627 = case shown="True" w1266 {
                tunnel: w1260 -> [w1272 w1282]
                tunnel: [w1272 w1281] -> w1265
                tunnel: w1264 -> [_ w1277]
                tunnel: w1263 -> [w1271 w1280]
                tunnel: [w1271 w1279] -> w1262
                tunnel: w1261 -> [_ w1278]
                frame False {
                }
                frame True {
                  w1273 = u8 0 ("Write Attribute")
                  w1274 = TRUE ("Bundle Element")
                  w1275 = FALSE ("Bundle Element")
                  n628 = Compound Arithmetic op=OR(w1278, w1277) -> (w1276:bool)
                  n629 = Bundle By Name(cluster=w1280, "halt now"=w1274, "changed"=w1274, "exit"=w1276) -> (w1279:T5)
                  n630 = property on="Signal Type" class="Ring (strict)"("Disabled"=w1273) -> ()  [unwired: 2 in, 2 out]
                  n631 = property on="Sel Channel" class="Ring (strict)"("Disabled"=w1273) -> ()  [unwired: 2 in, 2 out]
                  n632 = local write "start"(w1275) -> ()
                  n633 = Bundle By Name(cluster=w1282, "start"=w1275) -> (w1281:T14)
                  n634 = property on="Signal Path" class="Ring (strict)"("DisabledEnum"=w1273) -> ()  [unwired: 2 in, 2 out]
                }
              }
            }
            frame 2 {
              n635 = Unbundle By Name(w1284) -> ("Output Level(RMS)"=w1290:dbl)
              n636 = Not Equal?(x=w1290, y=w1289) -> (x != y?=w1283:bool)
              n637 = case shown="True" w1283 {
                tunnel: w1289 -> [_ w1300]
                tunnel: w1288 -> [w1292 w1313]
                tunnel: [w1292 w1312] -> w1287
                tunnel: w1286 -> [w1291 _]
                tunnel: [w1291 w1311] -> w1285
                tunnel: w1284 -> [_ w1310]
                frame False {
                }
                frame True {
                  n638 = local read "Vp Out"() -> (w1302:dbl)
                  n639 = Square Root(x=2.0) -> (sqrt(x)=w1305:dbl)
                  n640 = local read "Sensitivity"() -> (w1307:dbl)
                  n641 = Multiply(x=w1302, y=w1305) -> (x*y=w1306:dbl)
                  n642 = local read "Signal Type"() -> (w1309:i32)
                  n643 = Divide(x=w1306, y=2.0) -> (x/y=w1301:dbl)
                  n644 = Multiply(x=w1301, y=w1307) -> (x*y=w1308:dbl)
                  n645 = Max & Min(x=w1300, y=w1308) -> (min(x,y)=w1294:dbl)  [unwired: 1 out]
                  n646 = case shown="2, 3" w1309 {
                    tunnel: w1294 -> [_ w1316]
                    frame 0, Default {
                    }
                    frame 2, 3 {
                      n647 = local read "Vp Out"() -> (w1319:dbl)
                      n648 = local read "noise"() -> (w1317:sgl[])
                      n649 = call "CRYScale Wave.vi"("Level Type"=u16 0, "Level"=w1316, "dB ref"=1.0, "Max"=w1319, "Wave"=w1317) -> ("Scaled Wave"=w1315:sgl[])  [unwired: 4 in, 2 out]
                      n650 = local write "Play noise"(w1315) -> ()
                    }
                  }
                  n651 = local write "Output Level(RMS)"(w1294) -> ()
                  n652 = local read "dB ref."() -> (w1298:dbl)
                  n653 = Less?(x=w1294, y=1e-05) -> (x < y?=w1296:bool)
                  n654 = call "CRYConversion dB-Lin.vi"("dB ref."=w1298, "Lin In"=w1294) -> ("Log Out"=w1299:dbl)  [unwired: 4 in, 3 out]
                  n655 = Select(t=-1000.0, s=w1296, f=w1299) -> (s? t:f=w1293:dbl)
                  n656 = local write "wav level"(w1294) -> ()
                  n657 = Bundle By Name(cluster=w1310, "Output Level(RMS)"=w1294, "Output Level(dB)"=w1293) -> (w1311:T4)
                  n658 = Bundle By Name(cluster=w1313, "changed"=TRUE) -> (w1312:T5)
                  n659 = local write "dB"(w1293) -> ()
                }
              }
            }
            frame 3 {
              n660 = Unbundle By Name(w1326) -> ("Output Level(dB)"=w1329:dbl)
              n661 = Not Equal?(x=w1329, y=w1325) -> (x != y?=w1322:bool)
              n662 = case shown="True" w1322 {
                tunnel: w1325 -> [_ w1332]
                tunnel: w1328 -> [w1331 w1343]
                tunnel: [w1331 w1342] -> w1324
                tunnel: w1327 -> [w1330 _]
                tunnel: [w1330 w1341] -> w1323
                tunnel: w1326 -> [_ w1340]
                frame False {
                }
                frame True {
                  n663 = local read "dB ref."() -> (w1336:dbl)
                  n664 = call "CRYConversion dB-Lin.vi"("dB ref."=w1336, "Log In"=w1332) -> ("Lin Out"=w1338:dbl)  [unwired: 4 in, 3 out]
                  n665 = property on="Output Level(RMS)" class="Knob (strict)"() -> ("Maximum"=w1339:dbl)  [unwired: 2 in, 2 out]
                  n666 = Greater?(x=w1338, y=w1339) -> (0:w1337:bool)
                  n667 = case shown="True" w1337 {
                    tunnel: w1339 -> [_ w1353]
                    tunnel: [w1352 w1354] -> w1335
                    tunnel: w1332 -> [w1352 _]
                    tunnel: w1338 -> [w1351 _]
                    tunnel: [w1351 w1353] -> w1333
                    frame False {
                    }
                    frame True {
                      n668 = local read "dB ref."() -> (w1355:dbl)
                      n669 = call "CRYConversion dB-Lin.vi"("dB ref."=w1355, "Lin In"=w1353) -> ("Log Out"=w1354:dbl)  [unwired: 4 in, 3 out]
                      n670 = local write "dB"(w1354) -> ()
                    }
                  }
                  n671 = local read "Signal Type"() -> (w1334:i32)
                  n672 = case shown="2, 3" w1334 {
                    tunnel: w1333 -> [_ w1345]
                    frame 0, Default {
                    }
                    frame 2, 3 {
                      n673 = local read "Vp Out"() -> (w1349:dbl)
                      n674 = local read "noise"() -> (w1347:sgl[])
                      n675 = call "CRYScale Wave.vi"("Level Type"=u16 0, "Level"=w1345, "dB ref"=1.0, "Max"=w1349, "Wave"=w1347) -> ("Scaled Wave"=w1346:sgl[])  [unwired: 4 in, 2 out]
                      n676 = local write "Play noise"(w1346) -> ()
                    }
                  }
                  n677 = Bundle By Name(cluster=w1340, "Output Level(dB)"=w1335, "Output Level(RMS)"=w1333) -> (w1341:T4)
                  n678 = local write "Output Level(RMS)"(w1333) -> ()
                  n679 = local write "wav level"(w1333) -> ()
                  n680 = Bundle By Name(cluster=w1343, "changed"=TRUE) -> (w1342:T5)
                }
              }
            }
            frame 4 {
              n681 = Unbundle By Name(w1365) -> ("level lin/log"=w1367:bool)
              n682 = Unbundle By Name(w1362) -> ("wav init"=w1357:bool, "called"=w1356:bool)
              n683 = Exclusive Or(1:w1363, 2:w1367) -> (0:w1366:bool)
              n684 = Or(x=w1366, y=w1357) -> (x .or. y?=w1364:bool)
              n685 = case shown="True" w1364 {
                tunnel: w1363 -> [_ w1373]
                tunnel: w1360 -> [w1368 w1372]
                tunnel: w1356 -> [_ w1371]
                tunnel: w1359 -> [_ w1370]
                tunnel: [w1368 w1369] -> w1358
                frame False {
                }
                frame True {
                  n686 = stacked-sequence {
                    tunnel: w1373 -> [w1374 w1377]
                    tunnel: w1372 -> [_ w1381]
                    tunnel: w1371 -> [_ w1383]
                    tunnel: w1370 -> [_ w1382]
                    tunnel: [_ w1380] -> w1369
                    frame #0 {
                      n687 = Boolean To (0,1)(Boolean=w1374) -> (0, 1=w1375:i16)
                      n688 = property on="Output Level(RMS)" class="Knob (strict)"("Scale.Mapping Mode"=w1375) -> ()  [unwired: 2 in, 2 out]
                    }
                    frame #1 {
                      n689 = local write "wav ol log"(w1377) -> ()
                      n690 = Not(x=w1383) -> (.not. x?=w1379:bool)
                      n691 = local read "wav level"() -> (w1378:dbl)
                      n692 = Select(t=w1378, s=w1379, f=w1382) -> (s? t:f=w1376:dbl)
                      n693 = Bundle By Name(cluster=w1381, "Output Level(RMS)"=w1376) -> (w1380:T14)
                      n694 = disable-structure shown="Disabled" {
                        disable-tunnel: w1376 -> [w1384 _]
                        frame Disabled {
                          n695 = local write "Output Level(RMS)"(w1384) -> ()
                        }
                        frame Enabled {
                        }
                      }
                    }
                  }
                }
              }
            }
            frame 5 {
              n696 = Unbundle By Name(w1386) -> ("wav init"=w1389:bool)
              n697 = Or(x=w1389, y=w1388) -> (x .or. y?=w1387:bool)
              n698 = case shown="True" w1387 {
                tunnel: w1391 -> [_ w1403]
                tunnel: w1390 -> [_ w1402]
                tunnel: w1389 -> [_ w1399]
                tunnel: w1386 -> [w1395 w1397]
                tunnel: [w1393 w1396] -> w1385
                frame False {
                  n699 = Bundle By Name(cluster=w1395, "wav init"=FALSE) -> (w1393:T5)
                }
                frame True {
                  n700 = case shown="False" w1399 {
                    tunnel: [w1414 FALSE ("cancelled")] -> w1405
                    tunnel: [w1413 w1422] -> w1404
                    tunnel: [w1410 _] -> w1401
                    frame False {
                      n701 = flat-sequence {
                        tunnel: [w1419] -> w1410
                        tunnel: [w1416] -> w1409
                        frame #0 {
                          n702 = control-ref of="This VI"() -> (w1420:refnum<vi>)
                          n703 = property class="VI"(reference=w1420, "FP.Behavior"=T3."Floating" ("Front Panel Window:Behavior")) -> (reference out=w1419:refnum<vi>)  [unwired: 1 in, 1 out]
                          n704 = call "CRYGet Error Message.vi"("Error No"=1, "Kind"="Signal Generator") -> ("Message"=w1416:string)  [unwired: 4 in, 5 out]
                        }
                      }
                      n705 = global read "CRYMainGlobal.vi" "top path"() -> (w1411:path)
                      n706 = File Dialog(4:"Wave File" ("pattern label"), 6:"*.wav", 7:w1409, 11:w1411) -> (0:w1412:errorcluster, 1:w1414:bool, 3:w1413:path)  [unwired: 1 in, 3 out]
                      n707 = Unbundle(w1412) -> ()  [unwired: 3 out]
                    }
                    frame True {
                      n708 = local read "Wave path"() -> (w1423:string)
                      n709 = String To Path(string=w1423) -> (path=w1422:path)
                    }
                  }
                  n710 = case "canceled" shown="False" w1405 {
                    tunnel: w1404 -> [w1451 _]
                    tunnel: w1403 -> [w1447 _]
                    tunnel: w1402 -> [w1446 _]
                    tunnel: w1401 -> [w1445 w1460]
                    tunnel: [w1445 w1460] -> w1400
                    frame False {
                      n711 = Path To String(path=w1451) -> (string=w1443:string)
                      n712 = call "CRYGet Wave File Information.vi"("FileNameStr"=w1443) -> ("wave info"=w1440:T1, "wave data out"=w1428:i32[], "Error Output"=→"Error Output":errorcluster)  [unwired: 1 in, 11 out]
                      "wave info" <- w1440
                      n713 = local write "Wave path"(w1443) -> ()
                      n714 = Unbundle By Name(w1440) -> ("format str"=w1450:string, "Time Str"=w1449:string, "rms L"=→"rms L":dbl, "rms R"=→"rms R":dbl, "Channel Number"=w1427:u16)
                      n715 = local read "Sel Channel"() -> (w1426:u16)
                      n716 = call "CRYSplit Wave Data.vi"("sel channel"=w1426, "nChannels"=w1427, "wave data in"=w1428) -> ("wave data out"=w1425:i32[])  [unwired: 8 in]
                      n717 = local write "stereo"(w1450) -> ()
                      n718 = local write "Time"(w1449) -> ()
                      n719 = local write "wave data out"(w1425) -> ()
                      n720 = case shown="0, Default" w1447 {
                        tunnel: w1440 -> [w1453 w1455]
                        tunnel: [w1452 w1454] -> w1448
                        frame 0, Default {
                          n721 = Unbundle By Name(w1453) -> ("peak FSD"=w1452:dbl)
                        }
                        frame 1 {
                          n722 = Unbundle By Name(w1455) -> ("peak %FSD"=w1454:dbl)
                        }
                      }
                      n723 = case shown="0, Default" w1446 {
                        tunnel: w1440 -> [w1457 w1459]
                        tunnel: [w1456 w1458] -> w1444
                        frame 0, Default {
                          n724 = Unbundle By Name(w1457) -> ("rms FSD"=w1456:dbl)
                        }
                        frame 1 {
                          n725 = Unbundle By Name(w1459) -> ("rms %FSD"=w1458:dbl)
                        }
                      }
                      n726 = local write "Peak"(w1448) -> ()
                      n727 = local write "RMS"(w1444) -> ()
                      n728 = local read "Output Level(RMS)"() -> (w1438:dbl)
                      n729 = local read "Sensitivity"() -> (w1435:dbl)
                      n730 = local read "Vp Out"() -> (w1436:dbl)
                      n731 = Compound Arithmetic op=MULTIPLY(w1436, w1435) -> (w1433:dbl)
                      n732 = Divide(x=w1433, y=5.0) -> (x/y=w1432:dbl)
                      n733 = Greater?(x=w1438, y=w1432) -> (0:w1439:bool)
                      n734 = Select(t=w1432, s=w1439, f=w1438) -> (s? t:f=w1431:dbl)
                      n735 = property on="Output Level(RMS)" class="Knob (strict)"("Maximum"=w1432, "Scale.Maximum"=w1432, "Scale.Minimum"=0.0 ("Scale.Range:Minimum")) -> (error out=w1437:errorcluster)  [unwired: 2 in, 1 out]
                      n736 = local write "wav level"(w1431) -> ()
                      n737 = local write "Output Level(RMS)"(w1431) -> ()
                      n738 = case shown="No Error" w1437 {
                        frame No Error {
                        }
                        frame Error {
                        }
                      }
                    }
                    frame True {
                    }
                  }
                  n739 = Bundle By Name(cluster=w1397, "wav init"=FALSE) -> (w1396:T5)
                  n740 = case shown="False" w1399 {
                    tunnel: w1400 -> [w1406 _]
                    frame False {
                      n741 = property class="VI"(reference=w1406, "FP.Behavior"=T3."Floating" ("Front Panel Window:Behavior")) -> ()  [unwired: 1 in, 2 out]
                    }
                    frame True {
                    }
                  }
                }
              }
            }
            frame 6 {
              n742 = local read "wave info"() -> (w1462:T1)
              n743 = local read "wave info"() -> (w1463:T1)
              n744 = case shown="0, Default" w1465 {
                tunnel: w1462 -> [w1471 w1473]
                tunnel: [w1470 w1472] -> w1461
                frame 0, Default {
                  n745 = Unbundle By Name(w1471) -> ("peak FSD"=w1470:dbl)
                }
                frame 1 {
                  n746 = Unbundle By Name(w1473) -> ("peak %FSD"=w1472:dbl)
                }
              }
              n747 = case shown="0, Default" w1466 {
                tunnel: w1463 -> [w1475 w1477]
                tunnel: [w1474 w1476] -> w1464
                frame 0, Default {
                  n748 = Unbundle By Name(w1475) -> ("rms FSD"=w1474:dbl)
                }
                frame 1 {
                  n749 = Unbundle By Name(w1477) -> ("rms %FSD"=w1476:dbl)
                }
              }
              n750 = local write "RMS"(w1464) -> ()
              n751 = local write "Peak"(w1461) -> ()
            }
            frame 7 {
              n752 = Unbundle By Name(w1483) -> ("wav play mode"=w1485:i32)
              n753 = Not Equal?(x=w1485, y=w1479) -> (x != y?=w1478:bool)
              n754 = case shown="True" w1478 {
                tunnel: w1479 -> [_ w1496]
                tunnel: w1481 -> [w1486 w1494]
                tunnel: [w1486 w1493] -> w1480
                frame False {
                }
                frame True {
                  n755 = case shown="2" w1496 {
                    tunnel: [w1497 w1499 w1500] -> w1490
                    tunnel: u8 2 ("Write Attribute") -> [w1497 w1498 w1500]
                    tunnel: [w1497 w1498 w1501] -> w1489
                    tunnel: u8 0 ("Write Attribute") -> [_ w1499 w1501]
                    frame 0, Default {
                    }
                    frame 1 {
                    }
                    frame 2 {
                    }
                  }
                  n756 = property on="Duration" class="DigNum (strict)"("Disabled"=w1490) -> ()  [unwired: 2 in, 2 out]
                  n757 = property on="n times" class="DigNum (strict)"("Disabled"=w1489) -> ()  [unwired: 2 in, 2 out]
                  n758 = local write "start"(FALSE ("stop")) -> ()
                  n759 = Bundle By Name(cluster=w1494, "wav init"=FALSE, "halt now"=TRUE) -> (w1493:T5)
                }
              }
            }
            frame 8 {
              n760 = local read "Signal Path"() -> (w1506:i16)
              n761 = Unbundle By Name(w1505) -> ("Hardware"=w1507:i32)
              n762 = Not Equal?(x=w1507, y=w1506) -> (x != y?=w1502:bool)
              n763 = case shown="True" w1502 {
                tunnel: w1505 -> [w1509 w1548]
                tunnel: w1506 -> [_ w1544]
                tunnel: [w1509 w1542] -> w1504
                frame False {
                }
                frame True {
                  n764 = To Long Integer(number=w1544) -> (32bit integer=w1543:i32)
                  n765 = local read "Calibration in"() -> (w1522:string)
                  n766 = local read "Hardware in"() -> (w1523:string)
                  n767 = Bundle By Name(cluster=w1548, "changed"=TRUE, "Hardware"=w1543) -> (w1542:T5)
                  n768 = property on="Signal Path" class="Ring (strict)"() -> ("RingText.Text"=w1520:string)  [unwired: 2 in, 2 out]
                  n769 = call "CRYGet Hardware Info From Signal Type.vi"("Calibration In"=w1522, "Hardware In"=w1523, "Signal Type"=w1520, "In/Out?"=FALSE) -> ("Channel Info Out"=w1521:T12)  [unwired: 5 in, 2 out]
                  n770 = Unbundle By Name(w1521) -> ("ID"=w1545:i32, "Hardware Ch ID"=w1515:u8, "Sampling Rate (Hz)"=w1547:u32, "Bit Depth"=w1546:u32, "Vmax (V)"=w1519:dbl, "Audio Driver"=w1516:u16, "Device Name"=w1517:string)
                  n771 = call "CRYGet Current Calibration Info.vi"("Is Input?"=FALSE, "Signal Type Name"=w1520) -> ("Calibration All Cluster"=w1530:T7)  [unwired: 9 out]
                  n772 = local write "Output Device"(w1545) -> ()
                  n773 = local write "Channel Out"(w1515) -> ()
                  n774 = local write "BitDepth"(w1546) -> ()
                  n775 = local write "Fs"(w1547) -> ()
                  n776 = local write "Audio Driver"(w1516) -> ()
                  n777 = local write "Device Name"(w1517) -> ()
                  n778 = Unbundle By Name(w1530) -> ("EQ Curve"=w1540:T9, "Sens Curve"=w1538:T9)
                  n779 = Unbundle By Name(w1538) -> ("Curve"=w1536:cluster{"x":dbl, "y":dbl, "z":dbl}[], "Y unit"=w1511:string, "Y dB ref"=w1532:dbl)
                  n780 = Unbundle By Name(w1540) -> ("Curve"=w1539:cluster{"x":dbl, "y":dbl, "z":dbl}[])  [unwired: 1 out]
                  n781 = case shown="2" w1516 {
                    tunnel: w1515 -> [_ w1553]
                    frame 0, Default {
                      n782 = local read "Gen_Index"() -> (w1551:i32)
                      n783 = call "CRYUpdate Generator Index.vi"("Chn Idx"=-1, "Gen_Index"=w1551) -> ()  [unwired: 9 in]
                    }
                    frame 2 {
                      n784 = local read "Gen_Index"() -> (w1552:i32)
                      n785 = call "CRYUpdate Generator Index.vi"("Chn Idx"=w1553, "Gen_Index"=w1552) -> ()  [unwired: 9 in]
                    }
                  }
                  n786 = local write "Equalization Out"(w1539) -> ()
                  n787 = Reverse String(1:w1511) -> (0:w1514:string)
                  n788 = local write "buf_index"(u32 0 ("buf_index")) -> ()
                  n789 = Index Array(array=w1536) -> (element=w1537:cluster{"x":dbl, "y":dbl, "z":dbl})  [unwired: 1 in]
                  n790 = Match Pattern(string=w1514, regular expression="/" ("search char (-)")) -> (after substring=w1512:string)  [unwired: 1 in, 3 out]
                  n791 = Unbundle By Name(w1537) -> ("y"=w1533:dbl)
                  n792 = Reverse String(1:w1512) -> (0:w1510:string)
                  n793 = local write "unit2"(w1510) -> ()
                  n794 = global read "CRYCal Global.vi" "Calibrate"() -> (w1534:bool)
                  n795 = local read "Signal Type"() -> (w1535:i32)
                  n796 = case shown="False" w1534 {
                    tunnel: w1533 -> [w1555 _]
                    tunnel: w1532 -> [w1554 _]
                    tunnel: [w1555 w1557] -> w1527
                    tunnel: [w1554 1.0 ("y")] -> w1531
                    frame False {
                    }
                    frame True {
                      n797 = global read "CRYCal Global.vi" "Sens Out"() -> (w1557:dbl)
                    }
                  }
                  n798 = local write "Sensitivity"(w1527) -> ()
                  n799 = case shown="1, Default" w1535 {
                    tunnel: w1519 -> [_ w1569]
                    tunnel: w1531 -> [_ w1568]
                    tunnel: [w1560 w1566] -> w1526
                    tunnel: w1527 -> [w1562 _]
                    tunnel: [w1558 w1566] -> w1525
                    frame 2, 3 {
                      n800 = local read "Vp Out"() -> (w1564:dbl)
                      n801 = local read "Output Level(RMS)"() -> (w1561:dbl)
                      n802 = Compound Arithmetic op=MULTIPLY(w1564, w1562) -> (w1563:dbl)
                      n803 = Divide(x=w1563, y=5.0 ("x")) -> (x/y=w1560:dbl)
                      n804 = Greater?(x=w1561, y=w1560) -> (0:w1559:bool)
                      n805 = Select(t=w1560, s=w1559, f=w1561) -> (s? t:f=w1558:dbl)
                    }
                    frame 1, Default {
                      n806 = local read "RMS"() -> (w1567:dbl)
                      n807 = call "CRYConversion dB-Lin.vi"("dB ref."=w1568, "Log In"=w1567) -> ("Lin Out"=w1570:dbl)  [unwired: 4 in, 3 out]
                      n808 = Multiply(x=w1569, y=w1570) -> (x*y=w1566:dbl)
                    }
                  }
                  n809 = local write "Vp Out"(w1519) -> ()
                  n810 = local write "Output Level(RMS)"(w1525) -> ()
                  n811 = local write "dB ref."(w1531) -> ()
                  n812 = local write "wav level"(w1525) -> ()
                  n813 = property on="Output Level(RMS)" class="Knob (strict)"("Maximum"=w1526, "Scale.Maximum"=w1526, "Scale.Minimum"=0.0 ("Scale.Range:Minimum")) -> (error out=w1528:errorcluster)  [unwired: 2 in, 1 out]
                  n814 = case shown="No Error" w1528 {
                    frame No Error {
                    }
                    frame Error {
                    }
                  }
                }
              }
            }
            frame Default {
              n815 = Wait (ms)(milliseconds to wait=u32 10) -> ()  [unwired: 1 out]
              n816 = property on="Output Level(RMS)" class="Knob (strict)"() -> ("Scale.Range:Minimum"=w1573:dbl, "Scale.Range:Maximum"=w1572:dbl)  [unwired: 2 in, 2 out]
              n817 = local write "wav ol min"(w1573) -> ()
              n818 = local write "wav ol max"(w1572) -> ()
            }
          }
          n819 = Not(x=w1183) -> (.not. x?=w1184:bool)
        }
        n820 = Unbundle By Name(w781) -> ("changed"=w779:bool)
        n821 = And(x=w779, y=w780) -> (x .and. y?=w764:bool)
        n822 = Compound Arithmetic op=OR("start", w764) -> (w765:bool)
        n823 = case shown="True" w765 {
          tunnel: w788 -> [_ w815]
          tunnel: w787 -> [_ w824]
          tunnel: [w795 w809] -> w792
          tunnel: w781 -> [w794 w823]
          tunnel: [w794 w822] -> w790
          tunnel: w766 -> [_ w801]
          tunnel: w774 -> [_ w802]
          frame False {
            w795 = errorcluster {"status"=FALSE, "code"=0, "source"=""}  # no error
          }
          frame True {
            n824 = Unbundle By Name(w823) -> ("halt now"=w797:bool, "changed"=w806:bool)
            n825 = local read "Device Name"() -> (w798:string)
            n826 = local read "Output Device"() -> (w803:u32)
            n827 = local read "Audio Driver"() -> (w799:u16)
            n828 = local read "Channel Out"() -> (w816:u32)
            n829 = local read "Signal Type"() -> (w810:i32)
            n830 = local read "BitDepth"() -> (w817:u32)
            n831 = local read "Duration"() -> (w800:dbl)
            n832 = local read "n times"() -> (w821:i32)
            n833 = Not(x=w797) -> (.not. x?=w813:bool)
            n834 = local read "Fs"() -> (w818:u32)
            n835 = Boolean To (0,1)(Boolean=w806) -> (0, 1=w808:i16)
            n836 = Boolean To (0,1)(Boolean=w813) -> (0, 1=w814:i16)
            n837 = To Unsigned Long Integer(number=w821) -> (unsigned 32bit integer=w820:u32)
            n838 = To Unsigned Long Integer(number=w815) -> (unsigned 32bit integer=w812:u32)
            n839 = To Unsigned Byte Integer(number=w814) -> (unsigned 8bit integer=w811:u8)
            n840 = To Unsigned Byte Integer(number=w808) -> (unsigned 8bit integer=w807:u8)
            n841 = case shown="1" w810 {
              tunnel: w824 -> [w858 _]
              tunnel: w811 -> [w847 w1000]
              tunnel: [w855 w997] -> w819
              tunnel: [w856 w994] -> w804
              tunnel: w803 -> [w857 w1007]
              tunnel: w801 -> [w845 _]
              tunnel: w812 -> [w852 w1003]
              tunnel: w820 -> [w851 w1001]
              tunnel: [w854 w999] -> w796
              tunnel: w800 -> [w853 w1002]
              tunnel: w818 -> [w850 w1005]
              tunnel: w817 -> [w849 w1006]
              tunnel: w816 -> [w848 w1004]
              tunnel: w807 -> [w846 w998]
              tunnel: w799 -> [w844 w996]
              tunnel: w798 -> [w843 w995]
              tunnel: w797 -> [w842 w993]
              frame 1 {
                n842 = case shown="2" w844 {
                  tunnel: w858 -> [_ w992]
                  tunnel: w857 -> [_ w991]
                  tunnel: [w870 w990] -> w856
                  tunnel: [w872 w989] -> w855
                  tunnel: [w871 w988] -> w854
                  tunnel: w853 -> [w883 w987]
                  tunnel: w852 -> [w884 w986]
                  tunnel: w851 -> [w882 w985]
                  tunnel: w850 -> [w868 w984]
                  tunnel: w849 -> [w886 w983]
                  tunnel: w848 -> [w885 w982]
                  tunnel: w847 -> [_ w981]
                  tunnel: w846 -> [_ w975]
                  tunnel: w845 -> [w859 w974]
                  tunnel: w843 -> [w881 _]
                  tunnel: w842 -> [w873 _]
                  frame 2 {
                    n843 = local read "wave data out"() -> (w865:i32[])
                    n844 = local read "buf_index"() -> (w878:u32)
                    n845 = local read "asio start"() -> (w877:bool)
                    n846 = case shown="True" w877 {
                      selector: w877 -> [w962 w964]
                      tunnel: w881 -> [_ w973]
                      tunnel: w885 -> [_ w972]
                      tunnel: w868 -> [_ w971]
                      tunnel: w886 -> [_ w967]
                      tunnel: w882 -> [_ w969]
                      tunnel: [w962 w964] -> w876
                      tunnel: [w961 w963] -> w867
                      frame False {
                        n847 = local read "asio inited"() -> (w961:bool)
                      }
                      frame True {
                        n848 = local read "Gen_Index"() -> (w966:i32)
                        n849 = local write "nTime_Count"(w969) -> ()
                        n850 = call "CRYASIO Out & Init & Start.vi"("Bit Depth"=w967, "Sampling Rate"=w971, "Channel Index"=w972, "Device Name"=w973) -> ("bResult"=w963:bool, "Asio Opend Channel Index"=w970:u32)  [unwired: 6 in]
                        n851 = local write "asio start"(FALSE ("asio start")) -> ()
                        n852 = local write "Asio OCI"(w970) -> ()
                        n853 = local write "asio inited"(w963) -> ()
                        n854 = call "CRYSet Main Generator Array.vi"("Gen Idx"=w966) -> ("Is Main?"=w965:bool)  [unwired: 10 in]
                        n855 = local write "isMain"(w965) -> ()
                      }
                    }
                    n856 = Array Max & Min(array=w865) -> (max value=w864:i32)  [unwired: 3 out]
                    n857 = Divide(x=w865, y=w864) -> (x/y=w863:dbl[])
                    n858 = Square Root(x=2.0 ("y")) -> (sqrt(x)=w860:dbl)
                    n859 = Multiply(x=w859, y=w860) -> (x*y=w862:dbl)
                    n860 = Multiply(x=w863, y=w862) -> (x*y=w866:dbl[])
                    n861 = To Single Precision Float(number=w866) -> (single precision float=w880:sgl[])
                    n862 = case shown="1" w884 {
                      tunnel: w880 -> [w956 w960]
                      tunnel: [w955 w959] -> w879
                      tunnel: w878 -> [w954 w958]
                      tunnel: [w953 w957] -> w869
                      tunnel: w883 -> [w952 _]
                      tunnel: w868 -> [w951 _]
                      tunnel: w876 -> [_ _]
                      frame 1 {
                        n863 = call "CRYMake Asio Buffer.vi"("Fs"=w951, "Buffer Index"=w954, "Duration(s)"=w952, "Data Array"=w956) -> ("BufferIsEmpty?"=w955:bool, "Buf Data"=w953:sgl[])  [unwired: 6 in]
                      }
                      frame 0, Default {
                        n864 = call "CRYMake Asio Buffer.vi"("Buffer Index"=w958, "Data Array"=w960) -> ("BufferIsEmpty?"=w959:bool, "Buf Data"=w957:sgl[])  [unwired: 8 in]
                      }
                    }
                    n865 = local read "Gen_Index"() -> (w874:i32)
                    n866 = case shown="True" w867 {
                      tunnel: w879 -> [_ w900]
                      tunnel: w878 -> [_ w899]
                      tunnel: [TRUE w898] -> w870
                      tunnel: [w888 w897] -> w871
                      tunnel: [u32 10 ("return type") w896] -> w872
                      tunnel: w873 -> [_ w895]
                      tunnel: w884 -> [_ w894]
                      tunnel: w875 -> [_ w893]
                      tunnel: w885 -> [_ w892]
                      tunnel: w874 -> [_ w891]
                      frame False {
                        n867 = local read "asio finished"() -> (w888:bool)
                        n868 = Not(x=w888) -> (.not. x?=w887:bool)
                        n869 = local write "asio finished"(w887) -> ()
                      }
                      frame True {
                        n870 = case shown="False" w900 {
                          tunnel: w893 -> [w912 w924]
                          tunnel: w899 -> [w911 _]
                          tunnel: w894 -> [_ w921]
                          tunnel: [w907 w927] -> w898
                          tunnel: [w906 w926] -> w897
                          tunnel: [u32 0 ("return type") w925] -> w896
                          tunnel: w895 -> [w904 _]
                          tunnel: w892 -> [_ _]
                          tunnel: w891 -> [w902 w917]
                          frame False {
                            n871 = local read "BuffAmount"() -> (w901:u32)
                            n872 = local read "Asio OCI"() -> (w909:u32)
                            n873 = local read "isMain"() -> (w903:bool)
                            n874 = call "CRYASIO Play Buffer.vi"("Gen Idx"=w902, "is Main"=w903, "Limit"=w909, "Buffer Amount"=w901, "Buffer Index"=w911, "Data Array"=w912) -> ("Buffer Amount Out"=w908:u32, "Buffer Index Out"=w910:u32)  [unwired: 4 in]
                            n875 = local write "BuffAmount"(w908) -> ()
                            n876 = local write "buf_index"(w910) -> ()
                            n877 = local write "Buffer Amount"(w908) -> ()
                            n878 = case shown="True" w904 {
                              tunnel: [FALSE TRUE] -> w907
                              tunnel: [TRUE TRUE] -> w906
                              frame False {
                              }
                              frame True {
                              }
                            }
                          }
                          frame True {
                            n879 = local read "isMain"() -> (w918:bool)
                            n880 = local read "Asio OCI"() -> (w923:u32)
                            n881 = local read "BuffAmount"() -> (w920:u32)
                            n882 = call "CRYASIO Play Buffer.vi"("Gen Idx"=w917, "is Main"=w918, "Limit"=w923, "Buffer Amount"=w920, "Data Array"=w924) -> ("Buffer Amount Out"=w922:u32, "Buffer Index Out"=w919:u32)  [unwired: 5 in]
                            n883 = local write "BuffAmount"(w922) -> ()
                            n884 = case shown="2" w921 {
                              tunnel: [FALSE TRUE w939] -> w927
                              tunnel: [TRUE TRUE w938] -> w926
                              tunnel: [0 0 w937] -> w925
                              tunnel: w919 -> [_ _ _]
                              frame 0, Default {
                                n885 = local write "buf_index"(u32 0 ("buf_index")) -> ()
                              }
                              frame 1 {
                                n886 = local write "buf_index"(u32 0 ("buf_index")) -> ()
                              }
                              frame 2 {
                                n887 = local read "nTime_Count"() -> (w941:u32)
                                n888 = local write "buf_index"(u32 0 ("buf_index")) -> ()
                                n889 = Decrement(x=w941) -> (x-1=w940:u32)
                                n890 = local write "nTime_Count"(w940) -> ()
                                n891 = case shown="0" w940 {
                                tunnel: [TRUE FALSE] -> w939
                                tunnel: [TRUE TRUE] -> w938
                                tunnel: [1 0] -> w937
                                frame 0 {
                                }
                                frame 1, Default {
                                }
                                }
                              }
                            }
                          }
                        }
                      }
                    }
                    n892 = flat-sequence {
                      tunnel: w869 -> [w948]
                      tunnel: [w948] -> w875
                      frame #0 {
                        n893 = local read "Gen_Index"() -> (w950:i32)
                        n894 = call "CRYCheck Main Generator.vi"("Gen Idx"=w950) -> ("Is Main?"=w949:bool)  [unwired: 10 in]
                        n895 = local write "isMain"(w949) -> ()
                      }
                    }
                  }
                  frame 0, Default {
                    n896 = local read "ntaskID"() -> (w976:u32)
                    n897 = dll-call lib="D:/A_CRYSoundLab_Work/CRY6181/CRYSound.dll" fn="GVPlayWaveFile"("DeviceID"=w991, "WaveFileName"=w992, "SampleFreq"=w984, "BitDepth"=w983, "nChannels"=w982, "PlayMode"=w986, "Duration"=w987, "nTimes"=w985, "OutLevel"=w974, "startflag"=w981, "pauseflag"=u8 0, "changeflag"=w975, "ntaskID"=w976) -> ("return type"=w989:u32, "ntaskID"=w977:u32)  [unwired: 15 in, 2 out]
                    n898 = local write "ntaskID"(w977) -> ()
                    n899 = Not Equal?(x=w989, y=u32 0) -> (x != y?=w990:bool)
                    n900 = Less Or Equal?(x=w989, y=u32 1) -> (x <= y?=w988:bool)
                  }
                }
              }
              frame 2, 3, Default {
                n901 = case shown="2" w996 {
                  tunnel: w1007 -> [_ w1148]
                  tunnel: w1006 -> [w1028 w1147]
                  tunnel: w1005 -> [w1019 w1146]
                  tunnel: w1004 -> [w1015 w1145]
                  tunnel: w1003 -> [w1021 w1144]
                  tunnel: w1002 -> [w1020 w1143]
                  tunnel: w1001 -> [w1025 w1142]
                  tunnel: w1000 -> [_ w1141]
                  tunnel: [w1027 w1134] -> w994
                  tunnel: [w1026 w1133] -> w999
                  tunnel: w998 -> [_ w1132]
                  tunnel: [w1023 w1129] -> w997
                  tunnel: w995 -> [w1029 _]
                  tunnel: w993 -> [w1022 _]
                  frame 2 {
                    n902 = local read "buf_index"() -> (w1030:u32)
                    n903 = local read "asio start"() -> (w1024:bool)
                    n904 = local read "Sensitivity"() -> (w1011:dbl)
                    n905 = local read "Vp Out"() -> (w1012:dbl)
                    n906 = case shown="True" w1024 {
                      selector: w1024 -> [w1108 w1110]
                      tunnel: w1029 -> [_ w1119]
                      tunnel: w1015 -> [_ w1118]
                      tunnel: w1019 -> [_ w1117]
                      tunnel: w1028 -> [_ w1113]
                      tunnel: w1025 -> [_ w1115]
                      tunnel: [w1108 w1110] -> w1018
                      tunnel: [w1107 w1109] -> w1013
                      frame False {
                        n907 = local read "asio inited"() -> (w1107:bool)
                      }
                      frame True {
                        n908 = local read "Gen_Index"() -> (w1112:i32)
                        n909 = local write "nTime_Count"(w1115) -> ()
                        n910 = call "CRYASIO Out & Init & Start.vi"("Bit Depth"=w1113, "Sampling Rate"=w1117, "Channel Index"=w1118, "Device Name"=w1119) -> ("bResult"=w1109:bool, "Asio Opend Channel Index"=w1116:u32)  [unwired: 6 in]
                        n911 = local write "asio start"(FALSE ("asio start")) -> ()
                        n912 = local write "Asio OCI"(w1116) -> ()
                        n913 = local write "asio inited"(w1109) -> ()
                        n914 = call "CRYSet Main Generator Array.vi"("Gen Idx"=w1112) -> ("Is Main?"=w1111:bool)  [unwired: 10 in]
                        n915 = local write "isMain"(w1111) -> ()
                      }
                    }
                    n916 = Multiply(x=w1012, y=w1011) -> (x*y=w1008:dbl)
                    n917 = local read "Play noise"() -> (w1010:sgl[])
                    n918 = Divide(x=w1010, y=w1008) -> (x/y=w1009:dbl[])
                    n919 = To Single Precision Float(number=w1009) -> (single precision float=w1032:sgl[])
                    n920 = case shown="1" w1021 {
                      tunnel: w1032 -> [w1102 w1106]
                      tunnel: [w1101 w1105] -> w1031
                      tunnel: w1030 -> [w1100 w1104]
                      tunnel: [w1099 w1103] -> w1017
                      tunnel: w1020 -> [w1098 _]
                      tunnel: w1019 -> [w1097 _]
                      tunnel: w1018 -> [_ _]
                      frame 1 {
                        n921 = call "CRYMake Asio Buffer.vi"("Fs"=w1097, "Buffer Index"=w1100, "Duration(s)"=w1098, "Data Array"=w1102) -> ("BufferIsEmpty?"=w1101:bool, "Buf Data"=w1099:sgl[])  [unwired: 6 in]
                      }
                      frame 0, Default {
                        n922 = call "CRYMake Asio Buffer.vi"("Buffer Index"=w1104, "Data Array"=w1106) -> ("BufferIsEmpty?"=w1105:bool, "Buf Data"=w1103:sgl[])  [unwired: 8 in]
                      }
                    }
                    n923 = local read "Gen_Index"() -> (w1014:i32)
                    n924 = case shown="True" w1013 {
                      tunnel: w1031 -> [_ w1046]
                      tunnel: w1030 -> [_ w1045]
                      tunnel: [TRUE w1044] -> w1027
                      tunnel: [w1033 w1043] -> w1026
                      tunnel: [u32 10 ("return type") w1042] -> w1023
                      tunnel: w1022 -> [_ w1041]
                      tunnel: w1021 -> [_ w1040]
                      tunnel: w1016 -> [_ w1039]
                      tunnel: w1015 -> [_ w1038]
                      tunnel: w1014 -> [_ w1037]
                      frame False {
                        n925 = local read "asio finished"() -> (w1033:bool)
                        n926 = Not(x=w1033) -> (.not. x?=w1034:bool)
                        n927 = local write "asio finished"(w1034) -> ()
                      }
                      frame True {
                        n928 = case shown="False" w1046 {
                          tunnel: w1039 -> [w1058 w1070]
                          tunnel: w1045 -> [w1057 _]
                          tunnel: w1040 -> [_ w1067]
                          tunnel: [w1053 w1073] -> w1044
                          tunnel: [w1052 w1072] -> w1043
                          tunnel: [u32 0 ("return type") w1071] -> w1042
                          tunnel: w1041 -> [w1050 _]
                          tunnel: w1038 -> [_ _]
                          tunnel: w1037 -> [w1048 w1063]
                          frame False {
                            n929 = local read "BuffAmount"() -> (w1047:u32)
                            n930 = local read "Asio OCI"() -> (w1055:u32)
                            n931 = local read "isMain"() -> (w1049:bool)
                            n932 = call "CRYASIO Play Buffer.vi"("Gen Idx"=w1048, "is Main"=w1049, "Limit"=w1055, "Buffer Amount"=w1047, "Buffer Index"=w1057, "Data Array"=w1058) -> ("Buffer Amount Out"=w1054:u32, "Buffer Index Out"=w1056:u32)  [unwired: 4 in]
                            n933 = local write "BuffAmount"(w1054) -> ()
                            n934 = local write "buf_index"(w1056) -> ()
                            n935 = local write "Buffer Amount"(w1054) -> ()
                            n936 = case shown="False" w1050 {
                              tunnel: [FALSE TRUE] -> w1053
                              tunnel: [TRUE TRUE] -> w1052
                              frame False {
                              }
                              frame True {
                              }
                            }
                          }
                          frame True {
                            n937 = local read "isMain"() -> (w1064:bool)
                            n938 = local read "Asio OCI"() -> (w1069:u32)
                            n939 = local read "BuffAmount"() -> (w1066:u32)
                            n940 = call "CRYASIO Play Buffer.vi"("Gen Idx"=w1063, "is Main"=w1064, "Limit"=w1069, "Buffer Amount"=w1066, "Data Array"=w1070) -> ("Buffer Amount Out"=w1068:u32, "Buffer Index Out"=w1065:u32)  [unwired: 5 in]
                            n941 = local write "BuffAmount"(w1068) -> ()
                            n942 = case shown="1" w1067 {
                              tunnel: [FALSE TRUE w1085] -> w1073
                              tunnel: [TRUE TRUE w1084] -> w1072
                              tunnel: [0 0 w1083] -> w1071
                              tunnel: w1065 -> [_ _ _]
                              frame 0, Default {
                                n943 = local write "buf_index"(u32 0 ("buf_index")) -> ()
                              }
                              frame 1 {
                                n944 = local write "buf_index"(u32 0 ("buf_index")) -> ()
                              }
                              frame 2 {
                                n945 = local read "nTime_Count"() -> (w1087:u32)
                                n946 = local write "buf_index"(u32 0 ("buf_index")) -> ()
                                n947 = Decrement(x=w1087) -> (x-1=w1086:u32)
                                n948 = local write "nTime_Count"(w1086) -> ()
                                n949 = case shown="0" w1086 {
                                tunnel: [TRUE FALSE] -> w1085
                                tunnel: [TRUE TRUE] -> w1084
                                tunnel: [1 0] -> w1083
                                frame 0 {
                                }
                                frame 1, Default {
                                }
                                }
                              }
                            }
                          }
                        }
                      }
                    }
                    n950 = flat-sequence {
                      tunnel: w1017 -> [w1094]
                      tunnel: [w1094] -> w1016
                      frame #0 {
                        n951 = local read "Gen_Index"() -> (w1096:i32)
                        n952 = call "CRYCheck Main Generator.vi"("Gen Idx"=w1096) -> ("Is Main?"=w1095:bool)  [unwired: 10 in]
                        n953 = local write "isMain"(w1095) -> ()
                      }
                    }
                  }
                  frame 0, Default {
                    w1125 = 4194303.0  # 2^22 - 1
                    n954 = local read "Sensitivity"() -> (w1126:dbl)
                    n955 = local read "Vp Out"() -> (w1127:dbl)
                    n956 = local read "Play noise"() -> (w1122:sgl[])
                    n957 = Multiply(x=w1127, y=w1126) -> (x*y=w1121:dbl)
                    n958 = Divide(x=w1125, y=w1121) -> (x/y=w1124:dbl)
                    n959 = local read "Byte num"() -> (w1136:u32)
                    n960 = Multiply(x=w1122, y=w1124) -> (x*y=w1123:dbl[])
                    n961 = local read "ntaskID"() -> (w1131:u32)
                    n962 = To Single Precision Float(number=w1123) -> (single precision float=w1120:sgl[])
                    n963 = dll-call lib="D:/A_CRYSoundLab_Work/CRY6181/CRYSound.dll" fn="GVPlayMemory"("DeviceID"=w1148, "pSampleData"=w1120, "InSampleFreq"=w1146, "nInbitDepth"=u32 32, "nInChannels"=u32 1, "nInSampleLen"=w1136, "OutSampleFreq"=w1146, "nOutbitDepth"=w1147, "nOutChannels"=w1145, "PlayMode"=w1144, "Duration"=w1143, "nTimes"=w1142, "OutLevel"=1.0, "startflag"=w1141, "pauseflag"=u8 0, "changeflag"=w1132, "ntaskID"=w1131) -> ("return type"=w1129:u32, "ntaskID"=w1137:u32)  [unwired: 19 in, 2 out]
                    n964 = local write "ntaskID"(w1137) -> ()
                    n965 = Not Equal?(x=w1129, y=u32 0) -> (x != y?=w1134:bool)
                    n966 = Less Or Equal?(x=w1129, y=u32 1) -> (x <= y?=w1133:bool)
                  }
                }
              }
            }
            n967 = case shown="True" w804 {
              tunnel: w802 -> [_ w831]
              frame False {
              }
              frame True {
                n968 = local read "Audio Driver"() -> (w828:u16)
                n969 = local read "asio inited"() -> (w829:bool)
                n970 = local write "start"(FALSE ("start")) -> ()
                n971 = case shown="True" w831 {
                  frame False {
                  }
                  frame True {
                    n972 = local write "cancel2"(TRUE ("cancel2")) -> ()
                  }
                }
                n973 = local write "buf_index"(u32 0 ("buf_index")) -> ()
                n974 = Equal?(x=w828, y=u16 2) -> (x = y?=w826:bool)
                n975 = And(x=w826, y=w829) -> (x .and. y?=w825:bool)
                n976 = case shown="True" w825 {
                  frame False {
                    n977 = local write "asio finished"(FALSE ("asio finished")) -> ()
                  }
                  frame True {
                    n978 = local read "Channel Out"() -> (w837:u32)
                    n979 = local read "isMain"() -> (w835:bool)
                    n980 = local read "Gen_Index"() -> (w836:i32)
                    n981 = local read "Asio OCI"() -> (w838:u32)
                    n982 = local write "asio finished"(TRUE ("asio finished")) -> ()
                    n983 = local write "asio inited"(FALSE ("asio start")) -> ()
                    n984 = call "CRYASIO Close Cur Channel & Dev.vi"("Limit"=w838, "isInput?"=FALSE, "Channel Out"=w837) -> ()  [unwired: 9 in]
                    n985 = call "CRYClear Main Generator Array.vi"("isMain"=w835, "Gen Idx"=w836) -> ()  [unwired: 9 in, 1 out]
                  }
                }
              }
            }
            n986 = Bundle By Name(cluster=w823, "dll done"=w804, "halt now"=w804, "changed"=FALSE) -> (w822:T5)
            n987 = case shown="False" w796 {
              tunnel: w819 -> [w1154 _]
              tunnel: [w1162 w1167] -> w809
              tunnel: w802 -> [w1160 _]
              frame False {
                w1158 = errorcluster {FALSE, 0, ""}  # no error
                n988 = Equal?(x=w1154, y=u32 10) -> (x = y?=w1152:bool)
                n989 = Select(t=4 ("Error No"), s=w1152, f=3 ("Error No")) -> (s? t:f=w1149:i32)
                n990 = case shown="True" w1160 {
                  tunnel: [FALSE TRUE] -> w1159
                  frame False {
                  }
                  frame True {
                    n991 = local write "cancel2"(TRUE ("cancel2")) -> ()
                  }
                }
                n992 = call "CRYGet Error Message.vi"("Error No"=w1149, "Kind"="Signal Generator") -> ("Message"=w1157:string, "Window Title"=w1156:string)  [unwired: 4 in, 4 out]
                n993 = call "CRYMessage Dialog.vi"("Window Title"=w1156, "Message Content"=w1157) -> ()  [unwired: 8 in, 2 out]
                n994 = Bundle(cluster=w1158, w1159, w1154, "wave file player DLL") -> (w1162:errorcluster)
                n995 = local write "start"(FALSE ("start")) -> ()
              }
              frame True {
                w1167 = errorcluster {FALSE, 0, ""}  # no error
              }
            }
          }
        }
        n996 = Unbundle By Name(w792) -> ("status"=w782:bool)
        n997 = Unbundle By Name(w781) -> ("exit"=w783:bool)
        n998 = Not Or(1:w782, 2:w783) -> (0:w791:bool)
      }
    }
    n999 = local write "cont"(w249) -> ()
  }
  "error out" <- w5
  n1000 = local write "Canceled?"(w10) -> ()
  n1001 = stacked-sequence {
    tunnel: w10 -> [_ _ _]
    tunnel: w3 -> [_ _ _]
    frame #0 {
      n1002 = local read "Output Level(RMS)"() -> (w1585:dbl)
      n1003 = local read "Wave play mode"() -> (w1605:i32)
      n1004 = local read "Play Sine Wave:"() -> (w1582:i32)
      n1005 = property on="Output Level(RMS)" class="Knob (strict)"() -> ("Scale.Range:Minimum"=w1593:dbl, "Scale.Range:Maximum"=w1592:dbl)  [unwired: 2 in, 2 out]
      n1006 = property on="Frequency" class="Knob (strict)"() -> ("Scale.Range:Minimum"=w1602:dbl, "Scale.Range:Maximum"=w1601:dbl)  [unwired: 2 in, 2 out]
      n1007 = local read "Channel Out"() -> (w1587:u32)
      n1008 = local read "Signal Type"() -> (w1589:i32)
      n1009 = local read "Wave path"() -> (w1607:string)
      n1010 = local read "freq lin/log"() -> (w1591:bool)
      n1011 = local read "Duration(s)"() -> (w1599:dbl)
      n1012 = property on="Signal Path" class="Ring (strict)"() -> ("RingText.Text"=w1586:string)  [unwired: 2 in, 2 out]
      n1013 = local read "Frequency"() -> (w1606:dbl)
      n1014 = local read "wav ol log"() -> (w1600:bool)
      n1015 = local read "wav level"() -> (w1590:dbl)
      n1016 = local read "Duration"() -> (w1604:dbl)
      n1017 = local read "n times"() -> (w1603:i32)
      n1018 = local read "EQ"() -> (w1596:bool)
      n1019 = local write "Amp Out"(w1585) -> ()
      n1020 = local write "Freq Out"(w1606) -> ()
      n1021 = local read "Min (Hz)"() -> (w1598:dbl)
      n1022 = local read "Max(Hz)"() -> (w1597:dbl)
      n1023 = global read "CRYMisc vis settings global.vi" "Signal Gen'r settings"() -> (w1584:T11)
      n1024 = Bundle By Name(cluster=w1584, "gen'r mode"=w1589, "frequency"=w1606, "output level"=w1585, "wave path"=w1607, "wav play mode"=w1605, "duration"=w1604, "n times"=w1603, "wav level"=w1590, "channel"=w1587, "EQ"=w1596, "f knob high"=w1601, "f knob log"=w1591, "f knob low"=w1602, "ol knob high"=w1593, "ol knob log"=w1600, "ol knob low"=w1592, "Duration noise"=w1599, "Min freq noise"=w1598, "Max freq noise"=w1597, "Lin Display Prefs"="%#_6p", "dB Display Prefs"="%.1f", "Signal Type"=w1586, "Play Sine Wave"=w1582) -> (w1583:T11)
      n1025 = local read "asio inited"() -> (w1578:bool)
      n1026 = local read "Audio Driver"() -> (w1581:u16)
      n1027 = call "CRYFlatten Signal Generator.vi"("Signal Gen'r settings"=w1583) -> ("Flat Signal Gen'r settings"=→"Sigal generator setup Out":string)  [unwired: 10 out]
      n1028 = flat-sequence {
        tunnel: w1583 -> [w1613]
        frame #0 {
          n1029 = global write "CRYMisc vis settings global.vi" "Signal Gen'r settings"(w1613) -> ()
        }
        frame #1 {
        }
      }
      n1030 = Equal?(x=w1581, y=u16 2) -> (x = y?=w1579:bool)
      n1031 = And(x=w1579, y=w1578) -> (x .and. y?=w1577:bool)
      n1032 = case shown="True" w1577 {
        frame False {
        }
        frame True {
          n1033 = local read "Asio OCI"() -> (w1610:u32)
          n1034 = local read "Channel Out"() -> (w1612:u32)
          n1035 = local read "Gen_Index"() -> (w1608:i32)
          n1036 = local read "isMain"() -> (w1609:bool)
          n1037 = local write "asio inited"(FALSE ("asio start")) -> ()
          n1038 = call "CRYASIO Close Cur Channel & Dev.vi"("Limit"=w1610, "Channel Out"=w1612) -> ()  [unwired: 10 in]
          n1039 = call "CRYClear Main Generator Array.vi"("isMain"=w1609, "Gen Idx"=w1608) -> ()  [unwired: 9 in, 1 out]
        }
      }
    }
    frame #1 {
      n1040 = global read "CRYMisc vis settings global.vi" "Generator Index Array"() -> (w1616:T16)
      n1041 = local read "Gen_Index"() -> (w1618:i32)
      n1042 = for {
        tunnel: w1616 -> [w1626] mode=indexing
        tunnel: [w1625] -> w1615 mode=indexing
        n1043 = Unbundle By Name(w1626) -> ("Gen Idx"=w1625:i32)
      }
      n1044 = local read "close at end"() -> (w1624:bool)
      n1045 = local read "Manual"() -> (w1623:bool)
      n1046 = Search 1D Array(1D array=w1615, element=w1618) -> (index of element=w1614:i32)  [unwired: 1 in]
      n1047 = case shown="False" w1623 {
        frame False {
          n1048 = call "CRYSave Virtual Data.vi"() -> ()  [unwired: 1 in, 11 out]
        }
        frame True {
        }
      }
      n1049 = case shown="True" w1624 {
        frame False {
        }
        frame True {
          n1050 = property class="VI"("Front Panel Window:Open"=FALSE) -> ()  [unwired: 2 in, 2 out]
        }
      }
      n1051 = Delete From Array(array=w1616, index=w1614) -> (array with subset deleted=w1617:T16)  [unwired: 1 in, 1 out]
      n1052 = global write "CRYMisc vis settings global.vi" "Generator Index Array"(w1617) -> ()
      n1053 = global read "CRYMisc vis settings global.vi" "CloseAll Event"() -> (w1620:bool)
      n1054 = local read "Menu"() -> (w1622:bool)
      n1055 = Not(x=w1620) -> (.not. x?=w1619:bool)
      n1056 = And(x=w1622, y=w1619) -> (x .and. y?=w1621:bool)
      n1057 = case shown="True" w1621 {
        frame False {
        }
        frame True {
          n1058 = local read "VI nID"() -> (w1627:i32)
          n1059 = call "CRYOperator Process.vi"("VI ID"=w1627, "sAction"="Close", "sOperator Type"="OPERATOR_SIGGEN" ("sAction")) -> ()  [unwired: 8 in, 1 out]
        }
      }
    }
    frame #2 {
      n1060 = local write "StateOut"(TRUE ("StateOut")) -> ()
    }
  }
